vi "滑移力检测.vi"() -> ()   [LabVIEW 2020]
uses:
  <vilib>/Utility/config.llb/NI_LVConfig.lvlib
  Global_Variable/Global.vi
  Global_Variable/A131258.vi
  Database/Global1.vi
  <vilib>/addons/database/NI_Database_API.lvlib
  <vilib>/addons/database/Connection.llb/Conn Execute.vi
  <vilib>/addons/database/Recordset.llb/Rec Fetch Recordset Data (R).vi
  <vilib>/addons/database/Connection.llb/DB Tools Open Connec (String).vi
panel:
  out "Fdeviceid":string
  out "拉位移内最大压力追溯结果":bool
  out "压位移内最大压力追溯结果":bool
  out "USER_ID":string
  out "deviceid":string
  out "productid":string
  out "产品型号":string
  out "codeid":string
  out "联机模式":string
  out "用户权限":string
  out "用户名":string
  out "最小值下限":dbl format="%_4g"
  out "最小值上限":dbl format="%_4g"
  out "拉位移内最小压力(N)":dbl format="%_5g"
  out "压位移内最小压力(N)":dbl format="%_5g"
  in  "报表":string[][](table)=[["mm"], ["mm/s"]]
  in  "判定结果 3":bool[][](array[boolean])=[[TRUE]]
  out "拉力判定框内波动压力(N)":dbl format="%_5g"
  out "压力判定框内波动压力(N)":dbl format="%_5g"
  in  "选项卡控件 2":enum32{"滑移力曲线", "参数查看"}(tab)
  out "上序状态显示":string
  out "上序状态":bool
  in  "质量报警":bool
  in  "设备缺料":bool
  in  "设备故障":bool
  out "产品追溯码":string
  out "最大值下限":dbl format="%_4g"
  out "最大值上限":dbl format="%_4g"
  out "拉位移内最大压力(N)":dbl format="%_5g"
  out "压位移内最大压力(N)":dbl format="%_5g"
  out "合格指示灯":bool
  out "不合格指示灯":bool
  out "力位移曲线 3":cluster{dbl[], dbl[]}[](graph)
  in  "删除":bool
  in  "确定":bool
  in  "添加":bool
  in  "退出":bool
  in  "更新":bool
  in  "产品型号":string(combo)
  in  "选项卡控件 3":enum32{"工位参数", "产品管理", "用户管理"}(tab)
  in  "坐标轴参数":string[][](table)=[["mm"], ["mm/s"]]
  in  "判定框参数":string[][](table)=[["mm"], ["mm/s"]]
  in  "结果判定参数":string[][](table)=[["mm"], ["mm/s"]]
  in  "请输入添加的产品名称":string
  in  "请选择要删除的产品":string(combo)
  in  "进入用户管理":bool
  # "滑移力检测"
  # "上序状态："
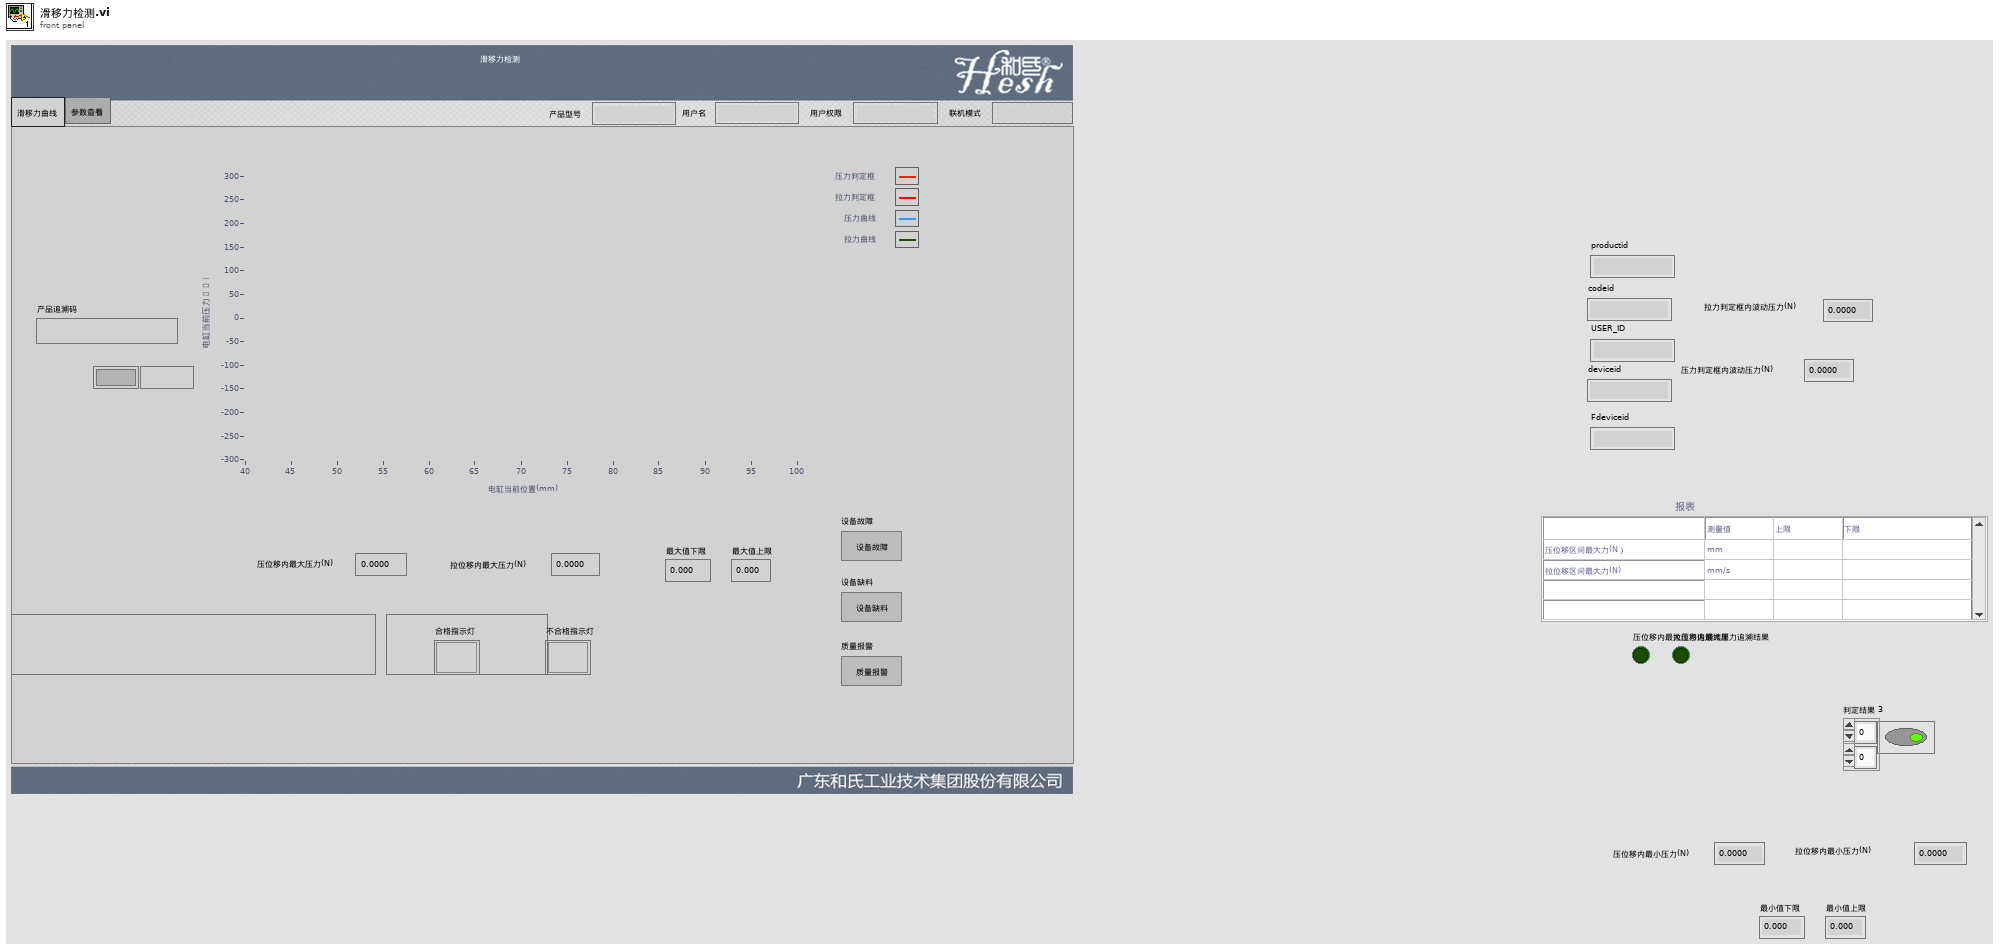
[diagram p1: front panel]
types:
  T1 = enum32{"Invalid", "Standard", "Closed", "Hidden", "Minimized", "Maximized"}
  T2 = cluster{"用户编号":string, "用户名":string, "用户密码(密文)":string, "用户权限":string}
  T3 = cluster{"设备名称":string, "用户名":string, "设备状态":enum16{"设备离线", "设备正常", "设备缺料", "设备故障", "质量报警"}, "附加信息":string}
  T4 = typedef "NI_LVConfig.lvlib/Config Data RefNum.ctl" = refnum<k1>
  T5 = cluster{i64, i64, string, "拉位移内最大压力(N)":dbl, "最大值下限":dbl, "最大值上限":dbl, string, string}
  T6 = cluster{i64, i64, string, "压位移内最大压力(N)":dbl, "最大值下限":dbl, "最大值上限":dbl, string, string}
  T7 = cluster{i64, i64, string, "拉位移内最大压力(N)":dbl, "最大值下限":dbl, "最大值上限":dbl, string, string}[]
  T8 = typedef "NI_Database_API.lvlib/Conn ObjectReference.ctl" = refnum<k1>
  T9 = cluster{i64, i64, "拉位移内最大压力(N)":dbl, "最大值下限":dbl, "最大值上限":dbl, string, string}
  T10 = cluster{i64, i64, i64, string, "result string":string}
  T11 = cluster{i64, i64, i64, string, "result string":string}[]
  T12 = typedef "NI_Database_API.lvlib/Rec ObjectReference.ctl" = refnum<k1>
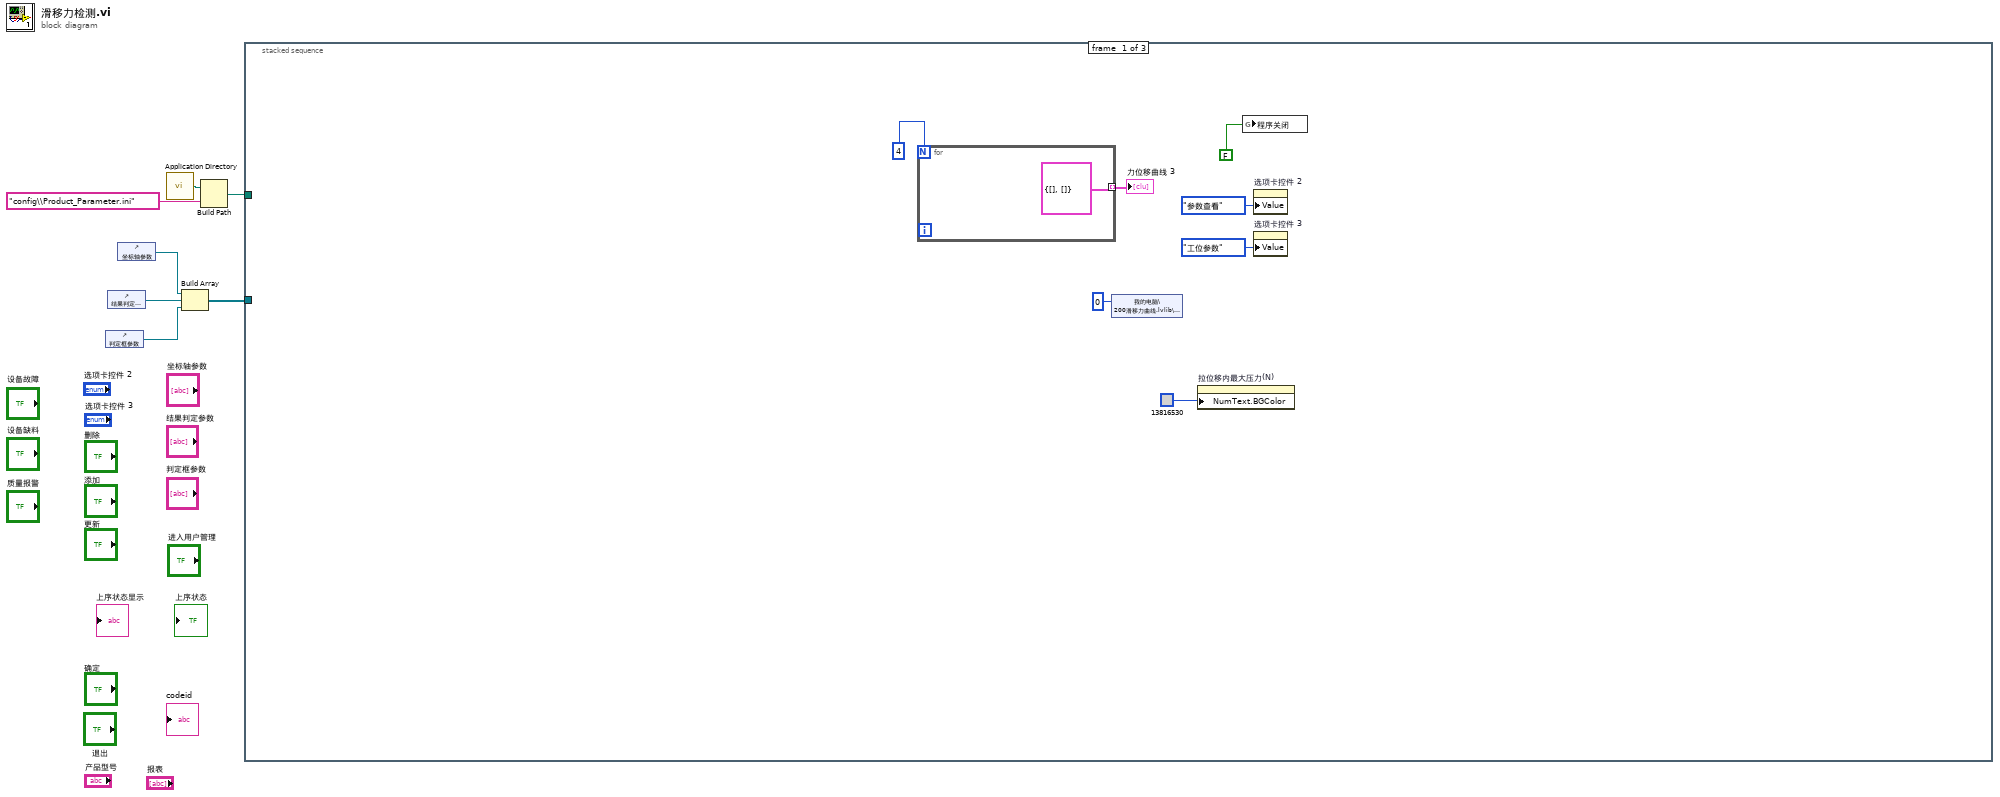
[diagram p0: block diagram]
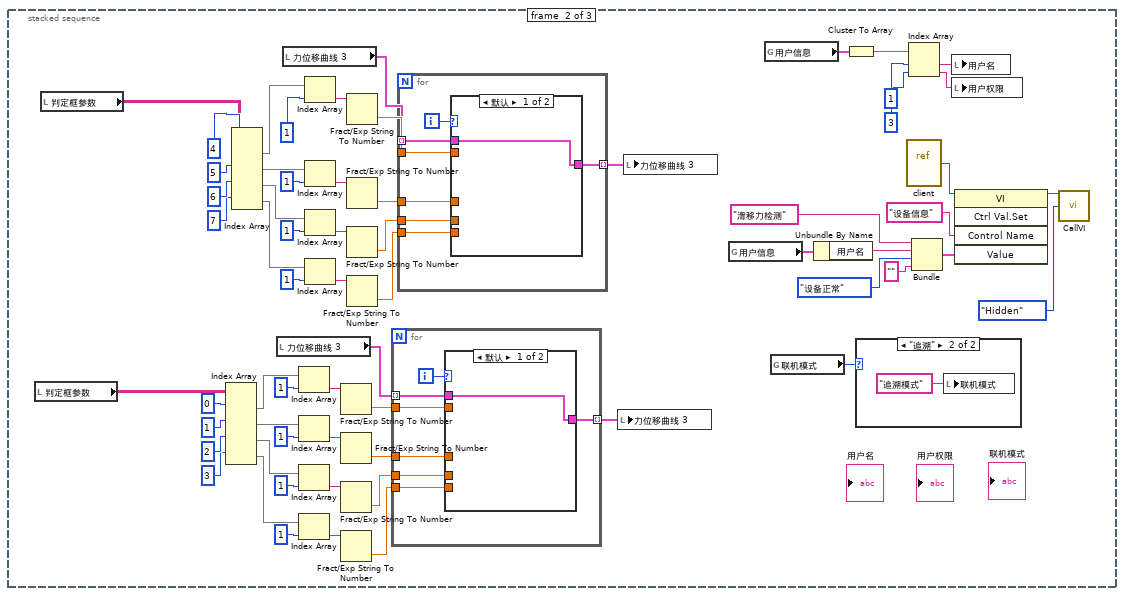
[diagram p2: hidden frame]
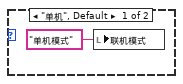
[diagram p3: hidden frame]
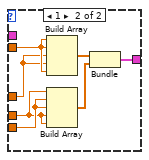
[diagram p4: hidden frame]
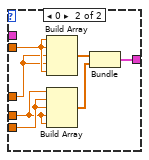
[diagram p5: hidden frame]
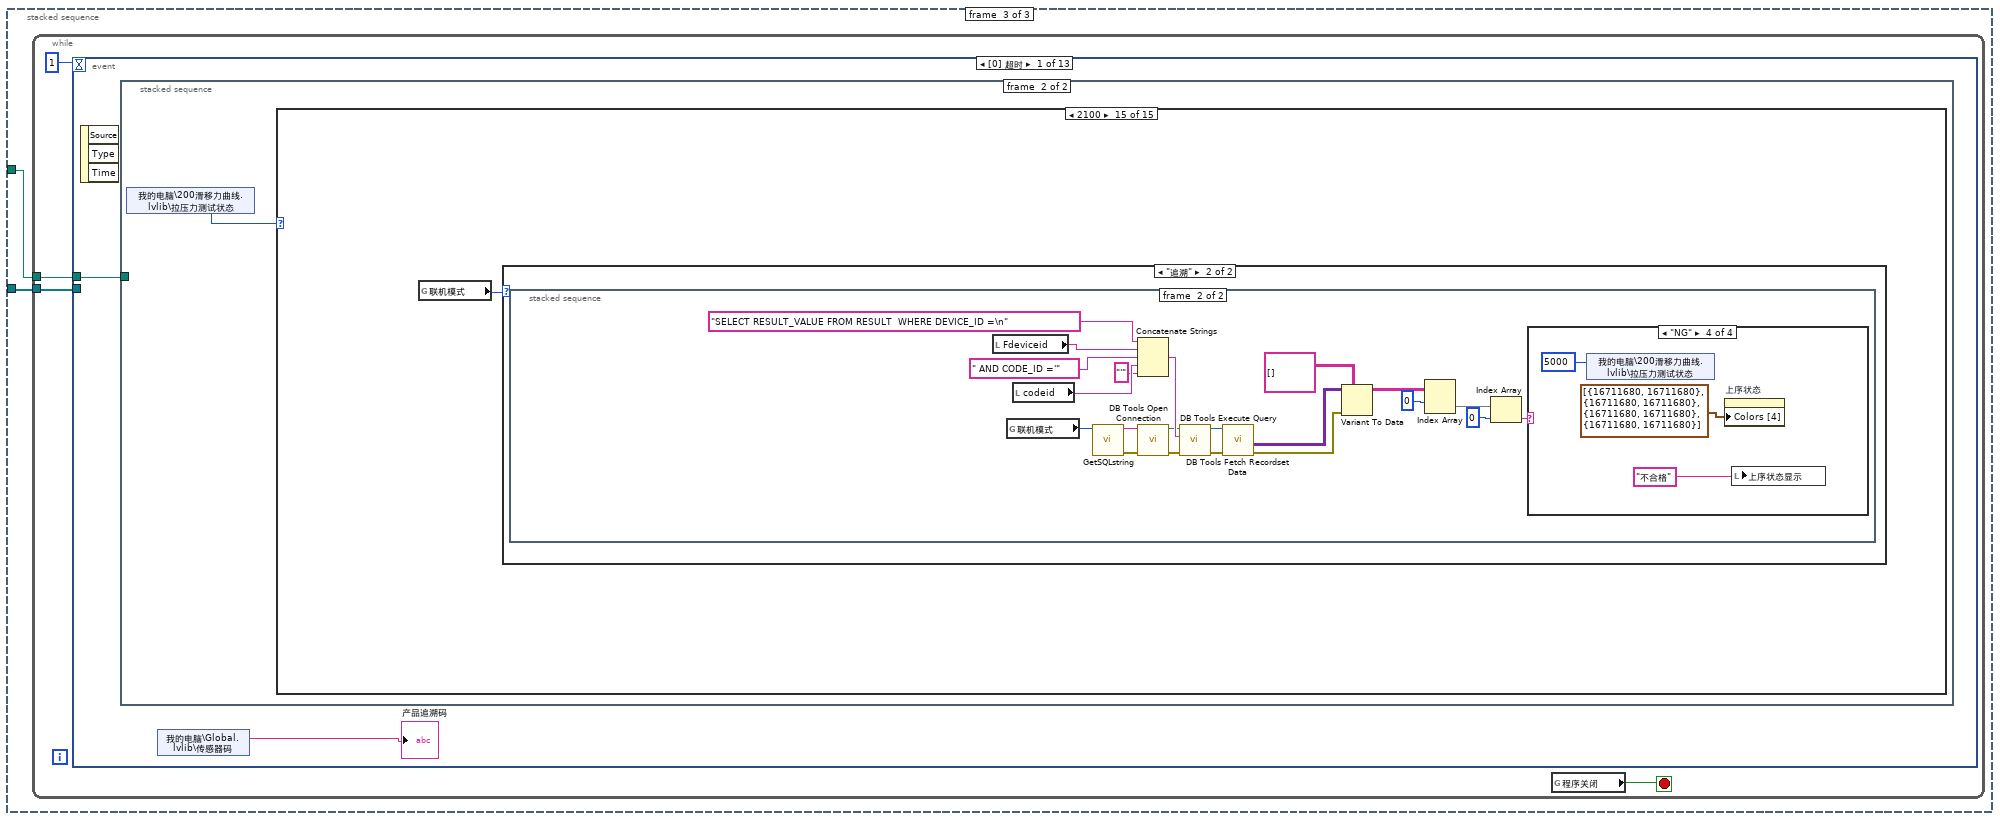
[diagram p6: hidden frame]
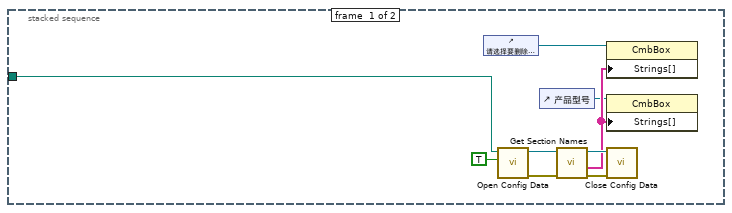
[diagram p7: hidden frame]
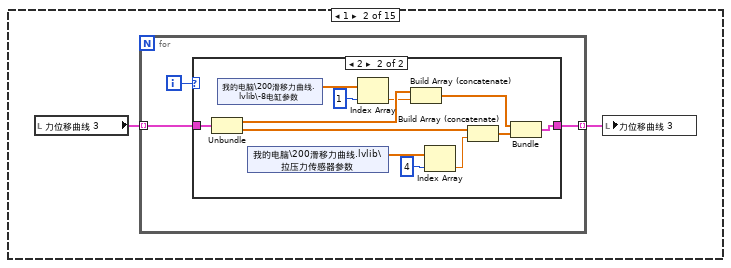
[diagram p9: hidden frame]
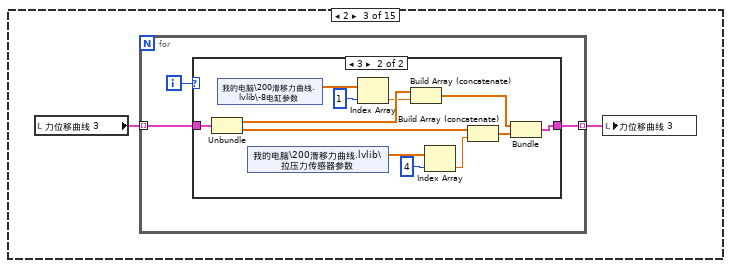
[diagram p11: hidden frame]
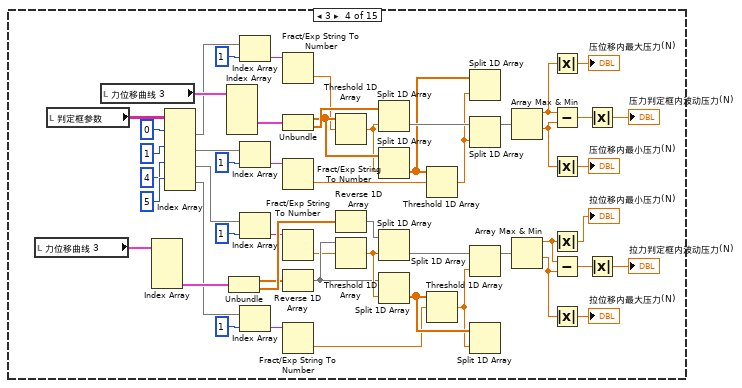
[diagram p13: hidden frame]
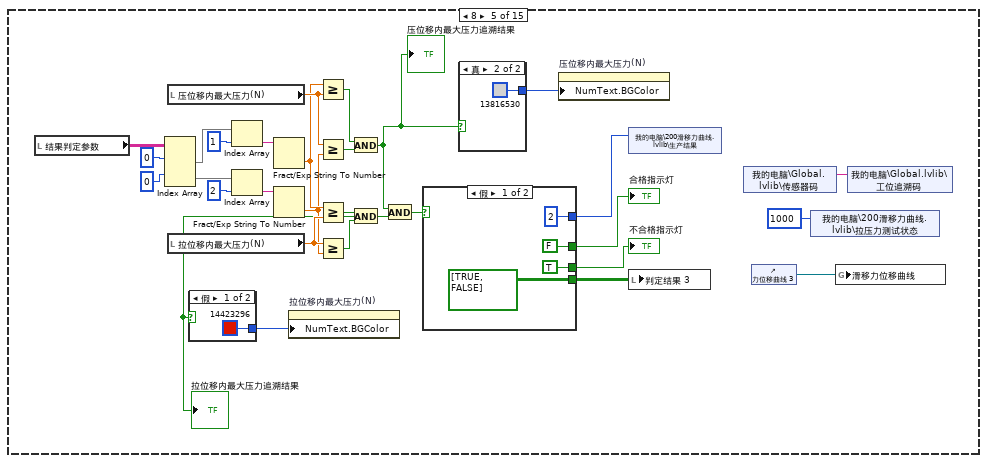
[diagram p14: hidden frame]
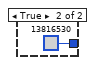
[diagram p15: hidden frame]
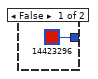
[diagram p16: hidden frame]
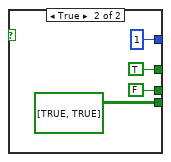
[diagram p17: hidden frame]
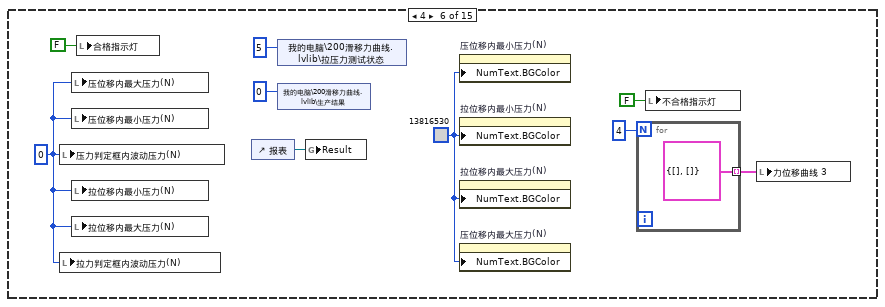
[diagram p18: hidden frame]
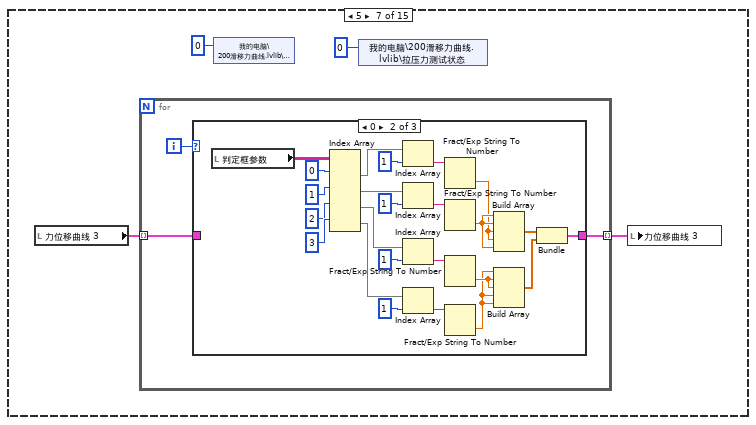
[diagram p19: hidden frame]
diagram:
  n1 = control-ref of="判定框参数"() -> (w1:refnum<vi>)
  n2 = control-ref of="结果判定参数"() -> (w2:refnum<vi>)
  n3 = control-ref of="坐标轴参数"() -> (w3:refnum<vi>)
  n4 = call <vilib>:"Application Directory.vi"() -> ("Application Directory"=w7:path)
  n5 = Build Array(w3, w2, w1) -> (w4:refnum<vi>[])
  n6 = Build Path(base path=w7, name or relative path="config\\Product_Parameter.ini" ("名称或相对路径")) -> (appended path=w5:path)
  n7 = stacked-sequence {
    tunnel: w5 -> [_ _ w112]
    tunnel: w4 -> [_ _ w111]
    frame #0 {
      n8 = for {
        N: 4 -> [_]
        tunnel: [cluster{dbl[], dbl[]} {[], []}] -> w13 mode=indexing
      }
      "力位移曲线 3" <- w13
      n9 = shared-variable "我的电脑\\200滑移力曲线.lvlib\\备用_1"(u16 0 ("备用_1")) -> ()  [unwired: 1 in, 1 out]
      n10 = property on="拉位移内最大压力(N)" class="DigNum (严格)"("NumText.BGColor"=u32 13816530) -> ()  [unwired: 2 in, 2 out]
      n11 = global write "Global.vi" "程序关闭"(FALSE ("程序关闭")) -> ()
      n12 = property on="选项卡控件 2" class="TabCtl (严格)"("Value"=enum32{"滑移力曲线", "参数查看"}."参数查看" ("选项卡控件 2")) -> ()  [unwired: 2 in, 2 out]
      n13 = property on="选项卡控件 3" class="TabCtl (严格)"("Value"=enum32{"工位参数", "产品管理"}."工位参数" ("选项卡控件 3")) -> ()  [unwired: 2 in, 2 out]
    }
    frame #1 {
      n14 = local read "判定框参数"() -> (w33:string[][])
      n15 = local read "判定框参数"() -> (w36:string[][])
      n16 = Index Array(array=w33, index (row) #1=0 ("索引 (行)"), index (row) #2=1 ("索引 (行)"), index (row) #3=2 ("索引 (行)"), index (row) #4=3 ("索引 (行)")) -> (element #1=w74:string[], element #2=w69:string[], element #3=w68:string[], element #4=w67:string[])  [unwired: 4 in]
      n17 = Index Array(array=w36, index (row) #1=4 ("索引 (行)"), index (row) #2=5 ("索引 (行)"), index (row) #3=6 ("索引 (行)"), index (row) #4=7 ("索引 (行)")) -> (element #1=w52:string[], element #2=w47:string[], element #3=w46:string[], element #4=w45:string[])  [unwired: 4 in]
      n18 = local read "力位移曲线 3"() -> (w57:cluster{dbl[], dbl[]}[])
      n19 = local read "力位移曲线 3"() -> (w35:cluster{dbl[], dbl[]}[])
      n20 = Index Array(array=w74, index=1 ("索引")) -> (element=w62:string)
      n21 = Index Array(array=w69, index=1 ("索引")) -> (element=w61:string)
      n22 = Index Array(array=w68, index=1 ("索引")) -> (element=w60:string)
      n23 = Index Array(array=w67, index=1 ("索引")) -> (element=w59:string)
      n24 = Index Array(array=w52, index=1 ("索引")) -> (element=w40:string)
      n25 = Index Array(array=w47, index=1 ("索引")) -> (element=w39:string)
      n26 = Index Array(array=w46, index=1 ("索引")) -> (element=w38:string)
      n27 = Index Array(array=w45, index=1 ("索引")) -> (element=w37:string)
      n28 = Fract/Exp String To Number(string=w62) -> (number=w66:dbl)  [unwired: 3 in, 1 out]
      n29 = Fract/Exp String To Number(string=w61) -> (number=w65:dbl)  [unwired: 3 in, 1 out]
      n30 = Fract/Exp String To Number(string=w60) -> (number=w63:dbl)  [unwired: 3 in, 1 out]
      n31 = Fract/Exp String To Number(string=w59) -> (number=w64:dbl)  [unwired: 3 in, 1 out]
      n32 = Fract/Exp String To Number(string=w40) -> (number=w44:dbl)  [unwired: 3 in, 1 out]
      n33 = Fract/Exp String To Number(string=w39) -> (number=w43:dbl)  [unwired: 3 in, 1 out]
      n34 = Fract/Exp String To Number(string=w38) -> (number=w41:dbl)  [unwired: 3 in, 1 out]
      n35 = Fract/Exp String To Number(string=w37) -> (number=w42:dbl)  [unwired: 3 in, 1 out]
      n36 = for {
        tunnel: [w102] -> w58 mode=indexing
        tunnel: w57 -> [w101] mode=indexing
        tunnel: w66 -> [w99]
        tunnel: w65 -> [w98]
        tunnel: w64 -> [w97]
        tunnel: w63 -> [w96]
        i -> [w100]
        n37 = case shown="默认" w100 {
          tunnel: [w103 w108] -> w102
          tunnel: w101 -> [w103 _]
          tunnel: w99 -> [_ w107]
          tunnel: w98 -> [_ w106]
          tunnel: w97 -> [_ w105]
          tunnel: w96 -> [_ w104]
          frame Default {
          }
          frame 0 {
            n38 = Build Array(w107, w107, w106, w106, w107) -> (w109:dbl[])
            n39 = Build Array(w104, w105, w105, w104, w104) -> (w110:dbl[])
            n40 = Bundle(w109, w110) -> (w108:cluster{dbl[], dbl[]})  [unwired: 1 in]
          }
        }
      }
      n41 = for {
        tunnel: [w87] -> w34 mode=indexing
        tunnel: w35 -> [w86] mode=indexing
        tunnel: w44 -> [w84]
        tunnel: w43 -> [w83]
        tunnel: w42 -> [w82]
        tunnel: w41 -> [w81]
        i -> [w85]
        n42 = case shown="默认" w85 {
          tunnel: [w88 w93] -> w87
          tunnel: w86 -> [w88 _]
          tunnel: w84 -> [_ w92]
          tunnel: w83 -> [_ w91]
          tunnel: w82 -> [_ w90]
          tunnel: w81 -> [_ w89]
          frame Default {
          }
          frame 1 {
            n43 = Build Array(w92, w92, w91, w91, w92) -> (w94:dbl[])
            n44 = Build Array(w89, w90, w90, w89, w89) -> (w95:dbl[])
            n45 = Bundle(w94, w95) -> (w93:cluster{dbl[], dbl[]})  [unwired: 1 in]
          }
        }
      }
      n46 = local write "力位移曲线 3"(w58) -> ()
      n47 = local write "力位移曲线 3"(w34) -> ()
      n48 = global read "Global1.vi" "用户信息"() -> (w23:T2)
      n49 = global read "Global1.vi" "用户信息"() -> (w32:T2)
      n50 = global read "Global1.vi" "联机模式"() -> (w26:enum16{"单机", "追溯"})
      n51 = Unbundle By Name(w23) -> ("用户名"=w22:string)
      n52 = Cluster To Array(cluster=w32) -> (array=w31:string[])
      n53 = case shown="\"追溯\"" w26 {
        frame "单机", Default {
          n54 = local write "联机模式"("单机模式" ("联机模式")) -> ()
        }
        frame "追溯" {
          n55 = local write "联机模式"("追溯模式" ("联机模式")) -> ()
        }
      }
      n56 = vi-ref "client.vi"() -> (w25:refnum<vi>)
      n57 = Index Array(array=w31, index #1=1 ("索引"), index #2=3 ("索引")) -> (element #1=w28:string, element #2=w27:string)
      n58 = Bundle("设备名称"="滑移力检测", "用户名"=w22, "设备状态"=enum16{"设备离线", "设备正常", "设备缺料", "设备故障", "质量报警"}."设备正常", "附加信息"="") -> (w21:T3)  [unwired: 1 in]
      n59 = local write "用户名"(w28) -> ()
      n60 = local write "用户权限"(w27) -> ()
      n61 = invoke class="VI" method="Ctrl Val.Set"(reference=w25, "Control Name"="设备信息" ("控件名"), "Value"=w21) -> (reference out=w24:refnum<vi>)  [unwired: 2 in, 4 out]
      n62 = call "CallVI.vi"("VI引用"=w24, "状态"=T1."Hidden") -> ()  [unwired: 11 in, 3 out]
    }
    frame #2 {
      n63 = while {
        tunnel: w112 -> [w115]
        tunnel: w111 -> [w114]
        stop <- w113 stop-if-true
        n64 = event shown="[0] 超时" {
          selector: _ -> [_ _ _ _ _ _ _ _ _ _ _ _ _]
          dyn-events: _ -> [_ _ _ _ _ _ _ _ _ _ _ _ _]
          timeout: 1 -> [_ _ _ _ _ _ _ _ _ _ _ _ _]
          tunnel: w115 -> [w118 w579 _ w747 w766 _ w777 _ _ _ _ _ _]
          tunnel: w114 -> [_ _ _ w746 w765 _ w776 _ _ _ _ _ _]
          event Timeout {
            n65 = event-data() -> ()  [unwired: 1 in, 3 out]
            n66 = stacked-sequence {
              tunnel: w118 -> [w119 _]
              frame #0 {
                n67 = control-ref of="请选择要删除的产品"() -> (w120:refnum<vi>)
                n68 = call <vilib>:"Open Config Data.vi"("create file if necessary (T)"=TRUE, "configuration file path"=w119) -> ("error out"=w124:errorcluster, "refnum"=w123:T4)  [unwired: 7 in, 1 out]
                n69 = control-ref of="产品型号"() -> (w121:refnum<vi>)
                n70 = call <vilib>:"Get Section Names.vi"("error in (no error)"=w124, "refnum"=w123) -> ("error out"=w126:errorcluster, "section names"=w122:string[], "refnum out"=w125:T4)  [unwired: 7 in]
                n71 = property on="属性节点" class="CmbBox"(reference=w120, "Strings[]"=w122) -> ()  [unwired: 1 in, 2 out]
                n72 = property on="属性节点" class="CmbBox"(reference=w121, "Strings[]"=w122) -> ()  [unwired: 1 in, 2 out]
                n73 = call <vilib>:"Close Config Data.vi"("error in (no error)"=w126, "refnum"=w125) -> ()  [unwired: 8 in, 2 out]
              }
              frame #1 {
                n74 = shared-variable "我的电脑\\200滑移力曲线.lvlib\\拉压力测试状态"() -> (w128:u16)  [unwired: 1 in, 1 out]
                n75 = case shown="2100" w128 {
                  frame 0, Default {
                  }
                  frame 1 {
                    n76 = local read "力位移曲线 3"() -> (w129:cluster{dbl[], dbl[]}[])
                    n77 = for {
                      tunnel: [w133] -> w130 mode=indexing
                      tunnel: w129 -> [w132] mode=indexing
                      i -> [w131]
                      n78 = case shown="2" w131 {
                        tunnel: [w134 w140] -> w133
                        tunnel: w132 -> [w134 w139]
                        frame Default {
                        }
                        frame 2 {
                          n79 = Unbundle(w139) -> (w144:dbl[], w143:dbl[])
                          n80 = shared-variable "我的电脑\\200滑移力曲线.lvlib\\-8电缸参数"() -> (w135:sgl[])  [unwired: 1 in, 1 out]
                          n81 = shared-variable "我的电脑\\200滑移力曲线.lvlib\\拉压力传感器参数"() -> (w136:sgl[])  [unwired: 1 in, 1 out]
                          n82 = Index Array(array=w135, index=1) -> (element=w137:sgl)
                          n83 = Build Array (concatenate)(w144, w137) -> (w142:dbl[])
                          n84 = Index Array(array=w136, index=4) -> (element=w138:sgl)
                          n85 = Build Array (concatenate)(w143, w138) -> (w141:dbl[])
                          n86 = Bundle(w142, w141) -> (w140:cluster{dbl[], dbl[]})  [unwired: 1 in]
                        }
                      }
                    }
                    n87 = local write "力位移曲线 3"(w130) -> ()
                  }
                  frame 2 {
                    n88 = local read "力位移曲线 3"() -> (w147:cluster{dbl[], dbl[]}[])
                    n89 = for {
                      tunnel: [w151] -> w148 mode=indexing
                      tunnel: w147 -> [w150] mode=indexing
                      i -> [w149]
                      n90 = case shown="3" w149 {
                        tunnel: [w152 w158] -> w151
                        tunnel: w150 -> [w152 w157]
                        frame Default {
                        }
                        frame 3 {
                          n91 = Unbundle(w157) -> (w162:dbl[], w161:dbl[])
                          n92 = shared-variable "我的电脑\\200滑移力曲线.lvlib\\-8电缸参数"() -> (w153:sgl[])  [unwired: 1 in, 1 out]
                          n93 = shared-variable "我的电脑\\200滑移力曲线.lvlib\\拉压力传感器参数"() -> (w154:sgl[])  [unwired: 1 in, 1 out]
                          n94 = Index Array(array=w153, index=1) -> (element=w155:sgl)
                          n95 = Build Array (concatenate)(w162, w155) -> (w160:dbl[])
                          n96 = Index Array(array=w154, index=4) -> (element=w156:sgl)
                          n97 = Build Array (concatenate)(w161, w156) -> (w159:dbl[])
                          n98 = Bundle(w160, w159) -> (w158:cluster{dbl[], dbl[]})  [unwired: 1 in]
                        }
                      }
                    }
                    n99 = local write "力位移曲线 3"(w148) -> ()
                  }
                  frame 3 {
                    n100 = local read "力位移曲线 3"() -> (w209:cluster{dbl[], dbl[]}[])
                    n101 = local read "判定框参数"() -> (w177:string[][])
                    n102 = local read "力位移曲线 3"() -> (w217:cluster{dbl[], dbl[]}[])
                    n103 = Index Array(array=w209) -> (element #4=w202:cluster{dbl[], dbl[]})  [unwired: 4 in, 3 out]
                    n104 = Index Array(array=w177, index (row) #1=0 ("索引 (行)"), index (row) #2=1 ("索引 (行)"), index (row) #3=4 ("索引 (行)"), index (row) #4=5 ("索引 (行)")) -> (element #1=w169:string[], element #2=w170:string[], element #3=w171:string[], element #4=w172:string[])  [unwired: 4 in]
                    n105 = Index Array(array=w217) -> (element #3=w203:cluster{dbl[], dbl[]})  [unwired: 4 in, 3 out]
                    n106 = Unbundle(w202) -> (w187:dbl[], w189:dbl[])
                    n107 = Index Array(array=w169, index=1 ("索引")) -> (element=w173:string)
                    n108 = Index Array(array=w170, index=1 ("索引")) -> (element=w174:string)
                    n109 = Index Array(array=w171, index=1 ("索引")) -> (element=w175:string)
                    n110 = Index Array(array=w172, index=1 ("索引")) -> (element=w176:string)
                    n111 = Fract/Exp String To Number(string=w173) -> (number=w168:dbl)  [unwired: 3 in, 1 out]
                    n112 = Unbundle(w203) -> (w215:dbl[], w216:dbl[])
                    n113 = Fract/Exp String To Number(string=w174) -> (number=w167:dbl)  [unwired: 3 in, 1 out]
                    n114 = Fract/Exp String To Number(string=w175) -> (number=w166:dbl)  [unwired: 3 in, 1 out]
                    n115 = Reverse 1D Array(array=w187) -> (reversed array=w186:dbl[])
                    n116 = Fract/Exp String To Number(string=w176) -> (number=w165:dbl)  [unwired: 3 in, 1 out]
                    n117 = Threshold 1D Array(2:w168, 3:w215) -> (0:w214:dbl)  [unwired: 1 in]
                    n118 = Reverse 1D Array(array=w189) -> (reversed array=w188:dbl[])
                    n119 = Threshold 1D Array(2:w166, 3:w186) -> (0:w208:dbl)  [unwired: 1 in]
                    n120 = Split 1D Array(array=w216, index=w214) -> (second subarray=w213:dbl[])  [unwired: 1 out]
                    n121 = Split 1D Array(array=w215, index=w214) -> (second subarray=w212:dbl[])  [unwired: 1 out]
                    n122 = Split 1D Array(array=w188, index=w208) -> (second subarray=w207:dbl[])  [unwired: 1 out]
                    n123 = Split 1D Array(array=w186, index=w208) -> (second subarray=w206:dbl[])  [unwired: 1 out]
                    n124 = Threshold 1D Array(2:w167, 3:w212) -> (0:w211:dbl)  [unwired: 1 in]
                    n125 = Threshold 1D Array(2:w165, 3:w206) -> (0:w205:dbl)  [unwired: 1 in]
                    n126 = Split 1D Array(array=w212, index=w211) -> ()  [unwired: 2 out]
                    n127 = Split 1D Array(array=w213, index=w211) -> (first subarray=w210:dbl[])  [unwired: 1 out]
                    n128 = Split 1D Array(array=w207, index=w205) -> (first subarray=w204:dbl[])  [unwired: 1 out]
                    n129 = Split 1D Array(array=w206, index=w205) -> ()  [unwired: 2 out]
                    n130 = Array Max & Min(array=w210) -> (max value=w193:dbl, min value=w191:dbl)  [unwired: 2 out]
                    n131 = Array Max & Min(array=w204) -> (max value=w201:dbl, min value=w199:dbl)  [unwired: 2 out]
                    n132 = Absolute Value(x=w193) -> (abs(x)=→"压位移内最大压力(N)":dbl)
                    n133 = Subtract(x=w193, y=w191) -> (x-y=w195:dbl)
                    n134 = Absolute Value(x=w191) -> (abs(x)=→"压位移内最小压力(N)":dbl)
                    n135 = Absolute Value(x=w201) -> (abs(x)=→"拉位移内最小压力(N)":dbl)
                    n136 = Subtract(x=w201, y=w199) -> (x-y=w197:dbl)
                    n137 = Absolute Value(x=w199) -> (abs(x)=→"拉位移内最大压力(N)":dbl)
                    n138 = Absolute Value(x=w195) -> (abs(x)=→"压力判定框内波动压力(N)":dbl)
                    n139 = Absolute Value(x=w197) -> (abs(x)=→"拉力判定框内波动压力(N)":dbl)
                  }
                  frame 8 {
                    n140 = local read "结果判定参数"() -> (w233:string[][])
                    n141 = Index Array(array=w233, index (row) #1=0 ("索引 (行)"), index (row) #2=0 ("索引 (行)")) -> (element #1=w229:string[], element #2=w230:string[])  [unwired: 2 in]
                    n142 = local read "压位移内最大压力(N)"() -> (w242:dbl)
                    n143 = local read "拉位移内最大压力(N)"() -> (w241:dbl)
                    n144 = Index Array(array=w229, index=1 ("索引")) -> (element=w231:string)
                    n145 = Index Array(array=w230, index=2 ("索引")) -> (element=w232:string)
                    n146 = Fract/Exp String To Number(string=w231) -> (number=w228:dbl)  [unwired: 3 in, 1 out]
                    n147 = Fract/Exp String To Number(string=w232) -> (number=w227:dbl)  [unwired: 3 in, 1 out]
                    n148 = Greater Or Equal?(x=w228, y=w242) -> (x >= y?=w246:bool)
                    n149 = Greater Or Equal?(x=w242, y=w227) -> (x >= y?=w245:bool)
                    n150 = Greater Or Equal?(x=w228, y=w241) -> (x >= y?=w244:bool)
                    n151 = Greater Or Equal?(x=w241, y=w227) -> (x >= y?=w243:bool)
                    n152 = And(x=w246, y=w245) -> (x .and. y?=w219:bool)
                    "压位移内最大压力追溯结果" <- w219
                    n153 = And(x=w244, y=w243) -> (x .and. y?=w218:bool)
                    "拉位移内最大压力追溯结果" <- w218
                    n154 = case shown="假" w218 {
                      tunnel: [u32 14423296 u32 13816530] -> w225
                      frame False {
                      }
                      frame True {
                      }
                    }
                    n155 = property on="拉位移内最大压力(N)" class="DigNum (严格)"("NumText.BGColor"=w225) -> ()  [unwired: 2 in, 2 out]
                    n156 = And(x=w219, y=w218) -> (x .and. y?=w220:bool)
                    n157 = case shown="假" w220 {
                      tunnel: [u16 2 ("生产结果") u16 1 ("生产结果")] -> w240
                      tunnel: [FALSE ("合格指示灯") TRUE ("合格指示灯")] -> w239
                      tunnel: [TRUE ("不合格指示灯") FALSE ("不合格指示灯")] -> w238
                      tunnel: [bool[][] [[TRUE, FALSE]] ("判定结果") bool[][] [[TRUE, TRUE]] ("判定结果")] -> w224
                      frame False {
                      }
                      frame True {
                      }
                    }
                    "不合格指示灯" <- w238
                    "合格指示灯" <- w239
                    n158 = case shown="真" w219 {
                      tunnel: [u32 14423296 u32 13816530] -> w226
                      frame False {
                      }
                      frame True {
                      }
                    }
                    n159 = property on="压位移内最大压力(N)" class="DigNum (严格)"("NumText.BGColor"=w226) -> ()  [unwired: 2 in, 2 out]
                    n160 = shared-variable "我的电脑\\200滑移力曲线.lvlib\\生产结果"(w240) -> ()  [unwired: 1 in, 1 out]
                    n161 = local write "判定结果 3"(w224) -> ()
                    n162 = shared-variable "我的电脑\\Global.lvlib\\传感器码"() -> (w223:string)  [unwired: 1 in, 1 out]
                    n163 = control-ref of="力位移曲线 3"() -> (w221:refnum<vi>)
                    n164 = shared-variable "我的电脑\\200滑移力曲线.lvlib\\拉压力测试状态"(u16 1000 ("拉压力测试状态")) -> ()  [unwired: 1 in, 1 out]
                    n165 = global write "A131258.vi" "滑移力位移曲线"(w221) -> ()
                    n166 = shared-variable "我的电脑\\Global.lvlib\\工位追溯码"(w223) -> ()  [unwired: 1 in, 1 out]
                  }
                  frame 4 {
                    w260 = u32 13816530
                    w264 = 0
                    n167 = local write "压力判定框内波动压力(N)"(w264) -> ()
                    n168 = local write "拉力判定框内波动压力(N)"(w264) -> ()
                    n169 = local write "压位移内最大压力(N)"(w264) -> ()
                    n170 = local write "压位移内最小压力(N)"(w264) -> ()
                    n171 = local write "拉位移内最小压力(N)"(w264) -> ()
                    n172 = local write "拉位移内最大压力(N)"(w264) -> ()
                    n173 = local write "合格指示灯"(FALSE ("合格指示灯")) -> ()
                    n174 = control-ref of="报表"() -> (w259:refnum<vi>)
                    n175 = shared-variable "我的电脑\\200滑移力曲线.lvlib\\拉压力测试状态"(5) -> ()  [unwired: 1 in, 1 out]
                    n176 = shared-variable "我的电脑\\200滑移力曲线.lvlib\\生产结果"(u16 0 ("生产结果")) -> ()  [unwired: 1 in, 1 out]
                    n177 = global write "Global.vi" "Result"(w259) -> ()
                    n178 = property on="压位移内最小压力(N)" class="DigNum (严格)"("NumText.BGColor"=w260) -> ()  [unwired: 2 in, 2 out]
                    n179 = property on="拉位移内最小压力(N)" class="DigNum (严格)"("NumText.BGColor"=w260) -> ()  [unwired: 2 in, 2 out]
                    n180 = property on="拉位移内最大压力(N)" class="DigNum (严格)"("NumText.BGColor"=w260) -> ()  [unwired: 2 in, 2 out]
                    n181 = property on="压位移内最大压力(N)" class="DigNum (严格)"("NumText.BGColor"=w260) -> ()  [unwired: 2 in, 2 out]
                    n182 = for {
                      N: 4 -> [_]
                      tunnel: [cluster{dbl[], dbl[]} {[], []}] -> w267 mode=indexing
                    }
                    n183 = local write "不合格指示灯"(FALSE ("不合格指示灯")) -> ()
                    n184 = local write "力位移曲线 3"(w267) -> ()
                  }
                  frame 5 {
                    n185 = local read "力位移曲线 3"() -> (w272:cluster{dbl[], dbl[]}[])
                    n186 = for {
                      tunnel: [w275] -> w271 mode=indexing
                      tunnel: w272 -> [w274] mode=indexing
                      i -> [w273]
                      n187 = case shown="0" w273 {
                        tunnel: [w276 w298 w301] -> w275
                        tunnel: w274 -> [w276 _ _]
                        frame Default {
                        }
                        frame 0 {
                          n188 = local read "判定框参数"() -> (w289:string[][])
                          n189 = Index Array(array=w289, index (row) #1=0 ("索引 (行)"), index (row) #2=1 ("索引 (行)"), index (row) #3=2 ("索引 (行)"), index (row) #4=3 ("索引 (行)")) -> (element #1=w281:string[], element #2=w282:string[], element #3=w283:string[], element #4=w284:string[])  [unwired: 4 in]
                          n190 = Index Array(array=w281, index=1 ("索引")) -> (element=w285:string)
                          n191 = Index Array(array=w282, index=1 ("索引")) -> (element=w286:string)
                          n192 = Index Array(array=w283, index=1 ("索引")) -> (element=w287:string)
                          n193 = Index Array(array=w284, index=1 ("索引")) -> (element=w288:string)
                          n194 = Fract/Exp String To Number(string=w285) -> (number=w279:dbl)  [unwired: 3 in, 1 out]
                          n195 = Fract/Exp String To Number(string=w286) -> (number=w280:dbl)  [unwired: 3 in, 1 out]
                          n196 = Fract/Exp String To Number(string=w287) -> (number=w278:dbl)  [unwired: 3 in, 1 out]
                          n197 = Fract/Exp String To Number(string=w288) -> (number=w277:dbl)  [unwired: 3 in, 1 out]
                          n198 = Build Array(w280, w280, w279, w279, w280) -> (w299:dbl[])
                          n199 = Build Array(w277, w278, w278, w277, w277) -> (w300:dbl[])
                          n200 = Bundle(w299, w300) -> (w298:cluster{dbl[], dbl[]})  [unwired: 1 in]
                        }
                        frame 1 {
                          n201 = local read "判定框参数"() -> (w322:string[][])
                          n202 = Index Array(array=w322, index (row) #1=4 ("索引 (行)"), index (row) #2=5 ("索引 (行)"), index (row) #3=6 ("索引 (行)"), index (row) #4=7 ("索引 (行)")) -> (element #1=w314:string[], element #2=w315:string[], element #3=w316:string[], element #4=w317:string[])  [unwired: 4 in]
                          n203 = Index Array(array=w314, index=1 ("索引")) -> (element=w318:string)
                          n204 = Index Array(array=w315, index=1 ("索引")) -> (element=w319:string)
                          n205 = Index Array(array=w316, index=1 ("索引")) -> (element=w320:string)
                          n206 = Index Array(array=w317, index=1 ("索引")) -> (element=w321:string)
                          n207 = Fract/Exp String To Number(string=w318) -> (number=w312:dbl)  [unwired: 3 in, 1 out]
                          n208 = Fract/Exp String To Number(string=w319) -> (number=w313:dbl)  [unwired: 3 in, 1 out]
                          n209 = Fract/Exp String To Number(string=w320) -> (number=w311:dbl)  [unwired: 3 in, 1 out]
                          n210 = Fract/Exp String To Number(string=w321) -> (number=w310:dbl)  [unwired: 3 in, 1 out]
                          n211 = Build Array(w313, w313, w312, w312, w313) -> (w323:dbl[])
                          n212 = Build Array(w310, w311, w311, w310, w310) -> (w324:dbl[])
                          n213 = Bundle(w323, w324) -> (w301:cluster{dbl[], dbl[]})  [unwired: 1 in]
                        }
                      }
                    }
                    n214 = shared-variable "我的电脑\\200滑移力曲线.lvlib\\备用_1"(u16 0 ("备用_1")) -> ()  [unwired: 1 in, 1 out]
                    n215 = shared-variable "我的电脑\\200滑移力曲线.lvlib\\拉压力测试状态"(0) -> ()  [unwired: 1 in, 1 out]
                    n216 = local write "力位移曲线 3"(w271) -> ()
                  }
                  frame 101 {
                    w327 = u32 13816530
                    w329 = 0.0 ("压力判定框内最大压力(N)")
                    w332 = FALSE ("合格指示灯")
                    n217 = shared-variable "我的电脑\\200滑移力曲线.lvlib\\备用_1"(u16 0 ("备用_1")) -> ()  [unwired: 1 in, 1 out]
                    n218 = local write "压位移内最大压力(N)"(w329) -> ()
                    n219 = local write "压位移内最小压力(N)"(w329) -> ()
                    n220 = local write "压力判定框内波动压力(N)"(w329) -> ()
                    n221 = local write "拉位移内最小压力(N)"(w329) -> ()
                    n222 = local write "拉位移内最大压力(N)"(w329) -> ()
                    n223 = local write "拉力判定框内波动压力(N)"(w329) -> ()
                    n224 = local write "合格指示灯"(w332) -> ()
                    n225 = local write "不合格指示灯"(w332) -> ()
                    n226 = property on="压位移内最大压力(N)" class="DigNum (严格)"("NumText.BGColor"=w327) -> ()  [unwired: 2 in, 2 out]
                    n227 = property on="压位移内最小压力(N)" class="DigNum (严格)"("NumText.BGColor"=w327) -> ()  [unwired: 2 in, 2 out]
                    n228 = property on="拉位移内最小压力(N)" class="DigNum (严格)"("NumText.BGColor"=w327) -> ()  [unwired: 2 in, 2 out]
                    n229 = property on="拉位移内最大压力(N)" class="DigNum (严格)"("NumText.BGColor"=w327) -> ()  [unwired: 2 in, 2 out]
                    n230 = shared-variable "我的电脑\\200滑移力曲线.lvlib\\生产结果"(u16 0 ("生产结果")) -> ()  [unwired: 1 in, 1 out]
                    n231 = shared-variable "我的电脑\\200滑移力曲线.lvlib\\拉压力测试状态"(0) -> ()  [unwired: 1 in, 1 out]
                    n232 = for {
                      N: 4 -> [_]
                      tunnel: [cluster{dbl[], dbl[]} {[], []}] -> w331 mode=indexing
                    }
                    n233 = local write "力位移曲线 3"(w331) -> ()
                  }
                  frame 1000 {
                    n234 = local read "压位移内最大压力(N)"() -> (w353:dbl)
                    n235 = local read "拉位移内最大压力(N)"() -> (w352:dbl)
                    n236 = local read "最大值上限"() -> (w350:dbl)
                    n237 = local read "最大值下限"() -> (w349:dbl)
                    n238 = local read "最大值上限"() -> (w348:dbl)
                    n239 = local read "最大值下限"() -> (w347:dbl)
                    n240 = Number To Fractional String(number=w353, precision (6)=i16 3 ("精度(6)")) -> (F-format string=w357:string)  [unwired: 2 in]
                    n241 = Number To Fractional String(number=w350, precision (6)=i16 3 ("精度(6)")) -> (F-format string=w356:string)  [unwired: 2 in]
                    n242 = Number To Fractional String(number=w349, precision (6)=i16 3 ("精度(6)")) -> (F-format string=w354:string)  [unwired: 2 in]
                    n243 = Number To Fractional String(number=w352, precision (6)=i16 3 ("精度(6)")) -> (F-format string=w351:string)  [unwired: 2 in]
                    n244 = Number To Fractional String(number=w348, precision (6)=i16 3 ("精度(6)")) -> (F-format string=w346:string)  [unwired: 2 in]
                    n245 = Number To Fractional String(number=w347, precision (6)=i16 3 ("精度(6)")) -> (F-format string=w345:string)  [unwired: 2 in]
                    n246 = Build Array(w357, w356, w354) -> (w355:string[])
                    n247 = Build Array(w351, w346, w345) -> (w335:string[])
                    n248 = Build Array(w355, w335) -> (w344:string[][])
                    n249 = local write "报表"(w344) -> ()
                    n250 = stacked-sequence {
                      frame #0 {
                        n251 = Wait (ms)(milliseconds to wait=u32 500 ("等待时间（毫秒）")) -> ()  [unwired: 1 out]
                        n252 = call "浮动通知.vi"("通知内容"="报表生成中" ("Status")) -> ()  [unwired: 11 in]
                      }
                      frame #1 {
                      }
                    }
                    n253 = control-ref of="报表"() -> (w343:refnum<vi>)
                    n254 = shared-variable "我的电脑\\200滑移力曲线.lvlib\\拉压力测试状态"(u16 1001 ("拉压力测试状态")) -> ()  [unwired: 1 in, 1 out]
                    n255 = shared-variable "我的电脑\\200滑移力曲线.lvlib\\备用_1"(u16 1 ("备用_1")) -> ()  [unwired: 1 in, 1 out]
                    n256 = global write "Global.vi" "Result"(w343) -> ()
                  }
                  frame 1001 {
                    n257 = shared-variable "我的电脑\\Global.lvlib\\工位追溯码"() -> (w364:string)  [unwired: 1 in, 1 out]
                    n258 = Wait (ms)(milliseconds to wait=u32 800 ("等待时间（毫秒）")) -> ()  [unwired: 1 out]
                    n259 = call "Report_A131258.vi"("文件重命名"=TRUE, "文件名称"=w364, "布尔数组"="判定结果 3") -> ()  [unwired: 8 in, 1 out]
                    n260 = shared-variable "我的电脑\\200滑移力曲线.lvlib\\拉压力测试状态"(u16 1002 ("备用1")) -> ()  [unwired: 1 in, 1 out]
                  }
                  frame 1002 {
                    n261 = global read "Global1.vi" "联机模式"() -> (w365:enum16{"单机", "追溯"})
                    n262 = case shown="\"追溯\"" w365 {
                      tunnel: w365 -> [_ w367]
                      frame "单机", Default {
                        n263 = shared-variable "我的电脑\\200滑移力曲线.lvlib\\拉压力测试状态"(u16 1003 ("备用1")) -> ()  [unwired: 1 in, 1 out]
                      }
                      frame "追溯" {
                        n264 = stacked-sequence {
                          tunnel: w367 -> [w368 _]
                          frame #0 {
                            n265 = local read "拉位移内最大压力追溯结果"() -> (w369:bool)
                            n266 = local read "压位移内最大压力追溯结果"() -> (w372:bool)
                            n267 = local read "拉位移内最大压力(N)"() -> (w382:dbl)
                            n268 = local read "压位移内最大压力(N)"() -> (w387:dbl)
                            n269 = local read "deviceid"() -> (w378:string)
                            n270 = local read "deviceid"() -> (w393:string)
                            n271 = local read "codeid"() -> (w381:string)
                            n272 = local read "codeid"() -> (w389:string)
                            n273 = local read "最大值下限"() -> (w383:dbl)
                            n274 = local read "最大值上限"() -> (w384:dbl)
                            n275 = local read "最大值下限"() -> (w386:dbl)
                            n276 = local read "最大值上限"() -> (w385:dbl)
                            n277 = case shown="假" w372 {
                              tunnel: ["NG" "OK"] -> w371
                              frame False {
                              }
                              frame True {
                              }
                            }
                            n278 = case shown="假" w369 {
                              tunnel: ["NG" "OK"] -> w370
                              frame False {
                              }
                              frame True {
                              }
                            }
                            n279 = Decimal String To Number(string=w378, default (0L)=i64 0 ("默认(0 I32)")) -> (number=w379:i64)  [unwired: 1 in, 1 out]
                            n280 = Decimal String To Number(string=w393, default (0L)=i64 0 ("默认(0 I32)")) -> (number=w391:i64)  [unwired: 1 in, 1 out]
                            n281 = Decimal String To Number(string=w381, default (0L)=i64 0 ("默认(0 I32)")) -> (number=w380:i64)  [unwired: 1 in, 1 out]
                            n282 = Decimal String To Number(string=w389, default (0L)=i64 0 ("默认(0 I32)")) -> (number=w390:i64)  [unwired: 1 in, 1 out]
                            n283 = Bundle(w379, w380, "拉位移内最大压力", "拉位移内最大压力(N)"=w382, "最大值下限"=w383, "最大值上限"=w384, "N", w370) -> (w373:T5)  [unwired: 1 in]
                            n284 = Bundle(w391, w390, "压位移内最大压力", "压位移内最大压力(N)"=w387, "最大值下限"=w386, "最大值上限"=w385, "N", w371) -> (w395:T6)  [unwired: 1 in]
                            n285 = Build Array(w395, w373) -> (w394:T7)
                            n286 = call "GetSQLstring.vi"("联机模式"=w368) -> ("错误输出"=w400:errorcluster, "连接字符串"=w401:string)  [unwired: 9 in]
                            n287 = call-poly <vilib>:"DB Tools Open Connection.vi"("error in (no error)"=w400, "connection information"=w401) -> ("error out"=w402:errorcluster, "connection reference"=w398:T8)  [unwired: 6 in]
                            n288 = for {
                              tunnel: w394 -> [w411] mode=indexing
                              tunnel: w398 -> [w409]
                              shift-right: [w407] -> w396
                              shift-left: w402 -> [w414]
                              w410 = string[] ["DEVICE_ID", "CODE_ID", "TEST_NAME", "TEST_VALUE", "TEST_VALUE_MIN", "TEST_VALUE_MAX", "TEST_VALUE_UNIT", "TEST_VALUE_RESULT"] ("columns")
                              w412 = "Test" ("table")
                              n289 = call <vilib>:"DB Tools Insert Data.vi"("data"=w411, "error in (no error)"=w414, "columns"=w410, "table"=w412, "connection reference"=w409) -> ("error out"=w413:errorcluster, "connection reference out"=w408:T8)  [unwired: 5 in]
                              n290 = case shown="错误" w413 {
                                selector: w413 -> [w415 w440]
                                tunnel: w410 -> [_ w437]
                                tunnel: w408 -> [w416 w422]
                                tunnel: w412 -> [_ w441]
                                tunnel: w411 -> [_ w431]
                                tunnel: [w416 w421] -> _
                                tunnel: [w415 w420] -> w407
                                frame No Error {
                                }
                                frame Error {
                                n291 = Delete From Array(array=w437, length=1 ("长度"), index=2 ("索引")) -> (array with subset deleted=w438:string[])  [unwired: 1 out]
                                n292 = call <vilib>:"Clear Errors.vi"("error in (no error)"=w440) -> ("error out"=w439:errorcluster)  [unwired: 5 in, 1 out]
                                n293 = Unbundle(w431) -> (w430:i64, w418:i64, w423:string, "拉位移内最大压力(N)"=w429:dbl, "最大值下限"=w428:dbl, "最大值上限"=w427:dbl, w426:string, w425:string)
                                n294 = Number To Decimal String(number=w418) -> (decimal integer string=w417:string)  [unwired: 1 in]
                                n295 = Bundle(w430, w418, "拉位移内最大压力(N)"=w429, "最大值下限"=w428, "最大值上限"=w427, w426, w425) -> (w424:T9)  [unwired: 1 in]
                                n296 = Concatenate Strings("WHERE TEST_NAME ='" ("condition"), w423, "'", "AND CODE_ID =" ("condition"), w417) -> (w433:string)
                                n297 = call <vilib>:"DB Tools Update Data.vi"("condition"=w433, "data"=w424, "error in (no error)"=w439, "columns"=w438, "table"=w441, "connection reference"=w422) -> ("error out"=w420:errorcluster, "connection reference out"=w421:T8)  [unwired: 4 in]
                                }
                              }
                            }
                            n298 = call <vilib>:"Simple Error Handler.vi"("error in (no error)"=w396) -> ()  [unwired: 4 in, 5 out]
                          }
                          frame #1 {
                            n299 = shared-variable "我的电脑\\200滑移力曲线.lvlib\\拉压力测试状态"(u16 1003 ("备用1")) -> ()  [unwired: 1 in, 1 out]
                          }
                        }
                      }
                    }
                  }
                  frame 1003 {
                    n300 = global read "Global1.vi" "联机模式"() -> (w443:enum16{"单机", "追溯"})
                    n301 = case shown="\"追溯\"" w443 {
                      tunnel: w443 -> [_ w446]
                      frame "单机", Default {
                        n302 = shared-variable "我的电脑\\200滑移力曲线.lvlib\\拉压力测试状态"(u16 0 ("备用1")) -> ()  [unwired: 1 in, 1 out]
                        n303 = shared-variable "我的电脑\\200滑移力曲线.lvlib\\备用_1"(u16 0 ("备用_1")) -> ()  [unwired: 1 in, 1 out]
                      }
                      frame "追溯" {
                        n304 = stacked-sequence {
                          tunnel: w446 -> [w447 _]
                          frame #0 {
                            n305 = shared-variable "我的电脑\\200滑移力曲线.lvlib\\生产结果"() -> (w449:u16)  [unwired: 1 in, 1 out]
                            n306 = case shown="2" w449 {
                              tunnel: ["" "OK" "NG"] -> w448
                              frame 0, Default {
                              }
                              frame 1 {
                              }
                              frame 2 {
                              }
                            }
                            n307 = Get Date/Time String(date format (0)=enum16{"short", "long", "abbreviated"}."short" ("日期格式(0)"), want seconds? (F)=FALSE ("需要秒？(F)")) -> (date string=w472:string, time string=w473:string)  [unwired: 1 in]
                            n308 = local read "USER_ID"() -> (w451:string)
                            n309 = local read "deviceid"() -> (w468:string)
                            n310 = local read "codeid"() -> (w470:string)
                            n311 = Concatenate Strings(w472, " " ("字符串"), w473) -> (w475:string)
                            n312 = Search and Replace String(replace all?=TRUE ("替换全部？(F)"), input string=w475, search string="/" ("替换字符串(\"\")"), replace string="-" ("替换字符串(\"\")")) -> (result string=w474:string)  [unwired: 4 in, 3 out]
                            n313 = Decimal String To Number(string=w468, default (0L)=i64 0 ("默认(0 I32)")) -> (number=w469:i64)  [unwired: 1 in, 1 out]
                            n314 = Decimal String To Number(string=w451, default (0L)=i64 0 ("默认(0 I32)")) -> (number=w450:i64)  [unwired: 1 in, 1 out]
                            n315 = Decimal String To Number(string=w470, default (0L)=i64 0 ("默认(0 I32)")) -> (number=w471:i64)  [unwired: 1 in, 1 out]
                            n316 = Bundle(w469, w450, w471, w448, "result string"=w474) -> (w466:T10)  [unwired: 1 in]
                            n317 = call "GetSQLstring.vi"("联机模式"=w447) -> ("错误输出"=w463:errorcluster, "连接字符串"=w462:string)  [unwired: 9 in]
                            n318 = Build Array(w466) -> (w467:T11)
                            n319 = call-poly <vilib>:"DB Tools Open Connection.vi"("error in (no error)"=w463, "connection information"=w462) -> ("error out"=w461:errorcluster, "connection reference"=w464:T8)  [unwired: 6 in]
                            n320 = for {
                              tunnel: w467 -> [w483] mode=indexing
                              tunnel: w464 -> [w481]
                              shift-right: [w479] -> w465
                              shift-left: w461 -> [w486]
                              w482 = string[] ["DEVICE_ID", "USER_ID", "CODE_ID", "RESULT_VALUE", "RESULT_TIME"] ("columns")
                              w484 = "Result" ("table")
                              n321 = call <vilib>:"DB Tools Insert Data.vi"("data"=w483, "error in (no error)"=w486, "columns"=w482, "table"=w484, "connection reference"=w481) -> ("error out"=w485:errorcluster, "connection reference out"=w480:T8)  [unwired: 5 in]
                              n322 = case shown="错误" w485 {
                                selector: w485 -> [w487 w508]
                                tunnel: w482 -> [_ w505]
                                tunnel: w480 -> [w488 w495]
                                tunnel: w484 -> [_ w509]
                                tunnel: w483 -> [_ w499]
                                tunnel: [w488 w494] -> _
                                tunnel: [w487 w493] -> w479
                                frame No Error {
                                }
                                frame Error {
                                n323 = Array Subset(array=w505, index=3 ("长度"), length=2 ("索引")) -> (w506:string[])
                                n324 = Unbundle(w499) -> (w490:i64, w491:i64, w498:string, "result string"=w497:string)  [unwired: 1 out]
                                n325 = Bundle(w498, "result string"=w497) -> (w496:cluster{string, "result string":string})  [unwired: 1 in]
                                n326 = Number To Decimal String(number=w491) -> (decimal integer string=w492:string)  [unwired: 1 in]
                                n327 = call <vilib>:"Clear Errors.vi"("error in (no error)"=w508) -> ("error out"=w507:errorcluster)  [unwired: 5 in, 1 out]
                                n328 = Number To Decimal String(number=w490) -> (decimal integer string=w489:string)  [unwired: 1 in]
                                n329 = Concatenate Strings("WHERE CODE_ID =" ("condition"), w492, "AND DEVICE_ID =", w489) -> (w501:string)
                                n330 = call <vilib>:"DB Tools Update Data.vi"("condition"=w501, "data"=w496, "error in (no error)"=w507, "columns"=w506, "table"=w509, "connection reference"=w495) -> ("error out"=w493:errorcluster, "connection reference out"=w494:T8)  [unwired: 4 in]
                                }
                              }
                            }
                            n331 = call <vilib>:"Simple Error Handler.vi"("error in (no error)"=w465) -> ()  [unwired: 4 in, 5 out]
                          }
                          frame #1 {
                            n332 = shared-variable "我的电脑\\200滑移力曲线.lvlib\\拉压力测试状态"(u16 0 ("备用1")) -> ()  [unwired: 1 in, 1 out]
                            n333 = shared-variable "我的电脑\\200滑移力曲线.lvlib\\备用_1"(u16 0 ("备用_1")) -> ()  [unwired: 1 in, 1 out]
                          }
                        }
                      }
                    }
                  }
                  frame 2000 {
                    n334 = stacked-sequence {
                      frame #0 {
                        n335 = Wait (ms)(milliseconds to wait=u32 300 ("等待时间（毫秒）")) -> ()  [unwired: 1 out]
                        n336 = shared-variable "我的电脑\\Global.lvlib\\传感器码"("" ("传感器码")) -> ()  [unwired: 1 in, 1 out]
                      }
                      frame #1 {
                        w518 = "请扫码！" ("通知内容")
                        n337 = call "浮动通知.vi"("通知内容"=w518) -> ()  [unwired: 11 in]
                        n338 = property on="上序状态" class="Bool (严格)"("Colors [4]"=cluster{u32, u32}[] [{11776947, 11776947}, {11776947, 11776947}, {11776947, 11776947}, {11776947, 11776947}]) -> ()  [unwired: 2 in, 2 out]
                        n339 = local write "上序状态显示"("" ("上序状态显示")) -> ()
                        n340 = call "输入框.vi"("提示信息"=w518) -> ("条形码输出"=w517:string)
                        n341 = shared-variable "我的电脑\\Global.lvlib\\传感器码"(w517) -> ()  [unwired: 1 in, 1 out]
                        n342 = shared-variable "我的电脑\\200滑移力曲线.lvlib\\拉压力测试状态"(u16 2001 ("备用1")) -> ()  [unwired: 1 in, 1 out]
                      }
                    }
                  }
                  frame 2001 {
                    n343 = shared-variable "我的电脑\\Global.lvlib\\传感器码"() -> (w521:string)  [unwired: 1 in, 1 out]
                    n344 = String Length(string=w521) -> (length=w520:i32)
                    n345 = Greater?(x=w520, y=4) -> (0:w522:bool)
                    n346 = case shown="真" w522 {
                      frame False {
                      }
                      frame True {
                        n347 = shared-variable "我的电脑\\200滑移力曲线.lvlib\\拉压力测试状态"(u16 2100 ("备用1")) -> ()  [unwired: 1 in, 1 out]
                      }
                    }
                  }
                  frame 2100 {
                    n348 = global read "Global1.vi" "联机模式"() -> (w524:enum16{"单机", "追溯"})
                    n349 = case shown="\"追溯\"" w524 {
                      frame "单机", Default {
                        n350 = shared-variable "我的电脑\\200滑移力曲线.lvlib\\拉压力测试状态"(u16 2002 ("备用1")) -> ()  [unwired: 1 in, 1 out]
                      }
                      frame "追溯" {
                        n351 = stacked-sequence {
                          frame #0 {
                            n352 = shared-variable "我的电脑\\Global.lvlib\\传感器码"() -> (w527:string)  [unwired: 1 in, 1 out]
                            n353 = local read "productid"() -> (w529:string)
                            n354 = global read "Global1.vi" "联机模式"() -> (w547:enum16{"单机", "追溯"})
                            n355 = call "GetSQLstring.vi"("联机模式"=w547) -> ("错误输出"=w545:errorcluster, "连接字符串"=w546:string)  [unwired: 9 in]
                            n356 = Concatenate Strings("SELECT CODE_ID  FROM CODE  WHERE CODE_SENSOR ='" ("字符串"), w527, "'" ("字符串"), " AND PRODUCT_ID='" ("字符串"), w529, "'" ("字符串")) -> (w544:string)
                            n357 = call-poly <vilib>:"DB Tools Open Connection.vi"("error in (no error)"=w545, "connection information"=w546) -> ("error out"=w538:errorcluster, "connection reference"=w539:T8)  [unwired: 6 in]
                            n358 = call-poly <vilib>:"DB Tools Execute Query.vi"("error in (no error)"=w538, "SQL query"=w544, "connection reference"=w539) -> ("error out"=w542:errorcluster, "recordset reference"=w543:T12)  [unwired: 5 in]
                            n359 = call-poly <vilib>:"DB Tools Fetch Recordset Data.vi"("error in (no error)"=w542, "recordset reference"=w543) -> ("error out"=w537:errorcluster, "recordset data"=w541:variant[][])  [unwired: 3 in, 1 out]
                            n360 = Variant To Data(error in=w537, type=string[][] [], Variant=w541) -> (data=w536:string[][])  [unwired: 1 out]
                            n361 = Index Array(array=w536, index (row)=0 ("索引 (行)")) -> (element=w534:string[])  [unwired: 1 in]
                            n362 = Index Array(array=w534, index=0 ("索引 (行)")) -> (element=w532:string)
                            n363 = local write "codeid"(w532) -> ()
                          }
                          frame #1 {
                            n364 = local read "Fdeviceid"() -> (w548:string)
                            n365 = global read "Global1.vi" "联机模式"() -> (w568:enum16{"单机", "追溯"})
                            n366 = local read "codeid"() -> (w550:string)
                            n367 = call "GetSQLstring.vi"("联机模式"=w568) -> ("错误输出"=w566:errorcluster, "连接字符串"=w567:string)  [unwired: 9 in]
                            n368 = Concatenate Strings("SELECT RESULT_VALUE FROM RESULT  WHERE DEVICE_ID =\n" ("table"), w548, " AND CODE_ID ='" ("字符串"), w550, "'" ("字符串")) -> (w565:string)
                            n369 = call-poly <vilib>:"DB Tools Open Connection.vi"("error in (no error)"=w566, "connection information"=w567) -> ("error out"=w559:errorcluster, "connection reference"=w560:T8)  [unwired: 6 in]
                            n370 = call-poly <vilib>:"DB Tools Execute Query.vi"("error in (no error)"=w559, "SQL query"=w565, "connection reference"=w560) -> ("error out"=w563:errorcluster, "recordset reference"=w564:T12)  [unwired: 5 in]
                            n371 = call-poly <vilib>:"DB Tools Fetch Recordset Data.vi"("error in (no error)"=w563, "recordset reference"=w564) -> ("error out"=w557:errorcluster, "recordset data"=w562:variant[][])  [unwired: 3 in, 1 out]
                            n372 = Variant To Data(error in=w557, type=string[][] [], Variant=w562) -> (data=w553:string[][])  [unwired: 1 out]
                            n373 = Index Array(array=w553, index (row)=0 ("索引 (行)")) -> (element=w555:string[])  [unwired: 1 in]
                            n374 = Index Array(array=w555, index=0 ("索引 (行)")) -> (element=w552:string)
                            n375 = case shown="\"NG\"" w552 {
                              frame "假", Default {
                              }
                              frame "" {
                                n376 = shared-variable "我的电脑\\200滑移力曲线.lvlib\\拉压力测试状态"(u16 5000 ("备用1")) -> ()  [unwired: 1 in, 1 out]
                                n377 = property on="上序状态" class="Bool (严格)"("Colors [4]"=cluster{u32, u32}[] [{16767232, 16767232}, {16767232, 16767232}, {16767232, 16767232}, {16767232, 16767232}]) -> ()  [unwired: 2 in, 2 out]
                                n378 = local write "上序状态显示"("漏序" ("上序状态显示")) -> ()
                              }
                              frame "OK" {
                                n379 = shared-variable "我的电脑\\200滑移力曲线.lvlib\\拉压力测试状态"(u16 2002 ("备用1")) -> ()  [unwired: 1 in, 1 out]
                                n380 = property on="上序状态" class="Bool (严格)"("Colors [4]"=cluster{u32, u32}[] [{6618880, 6618880}, {6618880, 6618880}, {6618880, 6618880}, {6618880, 6618880}]) -> ()  [unwired: 2 in, 2 out]
                                n381 = local write "上序状态显示"("合格" ("上序状态显示")) -> ()
                              }
                              frame "NG" {
                                n382 = shared-variable "我的电脑\\200滑移力曲线.lvlib\\拉压力测试状态"(u16 5000 ("备用1")) -> ()  [unwired: 1 in, 1 out]
                                n383 = property on="上序状态" class="Bool (严格)"("Colors [4]"=cluster{u32, u32}[] [{16711680, 16711680}, {16711680, 16711680}, {16711680, 16711680}, {16711680, 16711680}]) -> ()  [unwired: 2 in, 2 out]
                                n384 = local write "上序状态显示"("不合格" ("上序状态显示")) -> ()
                              }
                            }
                          }
                        }
                      }
                    }
                  }
                }
              }
            }
            n385 = shared-variable "我的电脑\\Global.lvlib\\传感器码"() -> (→"产品追溯码":string)  [unwired: 1 in, 1 out]
          }
          event "删除": Value Change {
            n386 = event-data() -> ("NewVal"=w578:bool)  [unwired: 1 in, 5 out]
            n387 = case shown="真" w578 {
              tunnel: w579 -> [_ w581]
              frame False {
              }
              frame True {
                n388 = Concatenate Strings("确认删除“", "请选择要删除的产品", "”吗？") -> (w583:string)
                n389 = Two Button Dialog(message=w583) -> (T button?=w582:bool)  [unwired: 2 in]
                n390 = case shown="真" w582 {
                  tunnel: w581 -> [_ w587]
                  tunnel: "请选择要删除的产品" -> [_ w586]
                  frame False {
                  }
                  frame True {
                    n391 = call <vilib>:"Open Config Data.vi"("configuration file path"=w587) -> ("error out"=w589:errorcluster, "refnum"=w592:T4)  [unwired: 8 in, 1 out]
                    n392 = call <vilib>:"Remove Section.vi"("section"=w586, "error in (no error)"=w589, "refnum"=w592) -> ("error out"=w591:errorcluster, "section exists?"=w588:bool, "refnum out"=w590:T4)  [unwired: 6 in]
                    n393 = case shown="假" w588 {
                      frame False {
                        n394 = One Button Dialog(message="删除失败！\n请确认产品存在！" ("消息")) -> ()  [unwired: 1 in, 1 out]
                      }
                      frame True {
                        n395 = One Button Dialog(message="删除成功！" ("消息")) -> ()  [unwired: 1 in, 1 out]
                      }
                    }
                    n396 = call <vilib>:"Close Config Data.vi"("error in (no error)"=w591, "refnum"=w590) -> ()  [unwired: 8 in, 2 out]
                  }
                }
              }
            }
          }
          event "确定": Value Change {
            n397 = event-data() -> ("NewVal"=w595:bool)  [unwired: 1 in, 5 out]
            n398 = case shown="真" w595 {
              frame False {
              }
              frame True {
                n399 = stacked-sequence {
                  seq-local: [w599 _ _ _ _ _ _] -> [_ _ _ _ _ _ _]
                  frame #0 {
                    n400 = global read "Global1.vi" "联机模式"() -> (w596:enum16{"单机", "追溯"})
                    n401 = case shown="\"追溯\"" w596 {
                      frame "单机", Default {
                      }
                      frame "追溯" {
                        n402 = local read "产品型号"() -> (w606:string)
                        n403 = call "Get_Device_ID.vi"() -> ("Device_ID"=→"deviceid":string)  [unwired: 10 in, 1 out]
                        n404 = call "GET_PRODUCT_ID.vi"("PRODFUCT_NAME"=w606) -> ("PRODUCT_ID"=w605:string)  [unwired: 10 in]
                        "productid" <- w605
                        n405 = call "查询前序设备.vi"("PRODUCT_ID"=w605) -> ("前序工位"=w604:string[])  [unwired: 10 in]
                        n406 = Index Array(array=w604, index=0 ("索引")) -> (element=→"Fdeviceid":string)
                      }
                    }
                    n407 = local read "产品型号"() -> (w598:string)
                    "产品型号" <- w598
                    n408 = shared-variable "我的电脑\\Global.lvlib\\产品型号"(w598) -> ()  [unwired: 1 in, 1 out]
                    n409 = String Subset(string=w598, offset (0)=u16 2 ("偏移量(0)"), length (rest)=u16 4 ("长度（剩余）")) -> (substring=w599:string)
                    n410 = property on="选项卡控件 2" class="TabCtl (严格)"("Value"=enum32{"滑移力曲线", "参数查看"}."滑移力曲线" ("选项卡控件 2")) -> ()  [unwired: 2 in, 2 out]
                    n411 = Fract/Exp String To Number(string=w599) -> ()  [unwired: 3 in, 2 out]
                  }
                  frame #1 {
                    n412 = local read "用户名"() -> (w609:string)
                    n413 = global read "Global1.vi" "联机模式"() -> (w615:enum16{"单机", "追溯"})
                    n414 = call "GetSQLstring.vi"("联机模式"=w615) -> ("错误输出"=w617:errorcluster, "连接字符串"=w616:string)  [unwired: 9 in]
                    n415 = call-poly <vilib>:"DB Tools Open Connection.vi"("error in (no error)"=w617, "connection information"=w616) -> ("error out"=w623:errorcluster, "connection reference"=w622:T8)  [unwired: 6 in]
                    n416 = Concatenate Strings("SELECT USER_ID FROM [User]  WHERE USER_NAME ='", w609, "'" ("字符串")) -> (w618:string)
                    n417 = call-poly <vilib>:"DB Tools Execute Query.vi"("error in (no error)"=w623, "SQL query"=w618, "connection reference"=w622) -> ("error out"=w620:errorcluster, "recordset reference"=w619:T12)  [unwired: 5 in]
                    n418 = call-poly <vilib>:"DB Tools Fetch Recordset Data.vi"("error in (no error)"=w620, "recordset reference"=w619) -> ("error out"=w624:errorcluster, "recordset data"=w621:variant[][])  [unwired: 3 in, 1 out]
                    n419 = Variant To Data(error in=w624, type=string[][] [], Variant=w621) -> (data=w625:string[][])  [unwired: 1 out]
                    n420 = Index Array(array=w625, index (row)=0 ("索引 (行)")) -> (element=w626:string[])  [unwired: 1 in]
                    n421 = Index Array(array=w626, index=0 ("索引 (行)")) -> (element=→"USER_ID":string)
                  }
                  frame #2 {
                    n422 = local read "坐标轴参数"() -> (w631:string[][])
                    n423 = Index Array(array=w631, index (row) #1=0 ("索引 (行)"), index (row) #2=1 ("索引 (行)"), index (row) #3=2 ("索引 (行)"), index (row) #4=3 ("索引 (行)")) -> (element #1=w643:string[], element #2=w638:string[], element #3=w637:string[], element #4=w636:string[])  [unwired: 4 in]
                    n424 = Index Array(array=w643, index=1 ("索引")) -> (element=w635:string)
                    n425 = Index Array(array=w638, index=1 ("索引")) -> (element=w634:string)
                    n426 = Index Array(array=w637, index=1 ("索引")) -> (element=w633:string)
                    n427 = Index Array(array=w636, index=1 ("索引")) -> (element=w632:string)
                    n428 = Fract/Exp String To Number(string=w635) -> (number=w630:dbl)  [unwired: 3 in, 1 out]
                    n429 = Fract/Exp String To Number(string=w634) -> (number=w629:dbl)  [unwired: 3 in, 1 out]
                    n430 = Fract/Exp String To Number(string=w633) -> (number=w628:dbl)  [unwired: 3 in, 1 out]
                    n431 = Fract/Exp String To Number(string=w632) -> (number=w627:dbl)  [unwired: 3 in, 1 out]
                    n432 = property on="力位移曲线 3" class="XYGraph (严格)"("XScale.Minimum"=w630) -> ()  [unwired: 2 in, 2 out]
                    n433 = property on="力位移曲线 3" class="XYGraph (严格)"("XScale.Maximum"=w629) -> ()  [unwired: 2 in, 2 out]
                    n434 = property on="力位移曲线 3" class="XYGraph (严格)"("YScale.Minimum"=w628) -> ()  [unwired: 2 in, 2 out]
                    n435 = property on="力位移曲线 3" class="XYGraph (严格)"("YScale.Maximum"=w627) -> ()  [unwired: 2 in, 2 out]
                  }
                  frame #3 {
                    n436 = local read "判定框参数"() -> (w657:string[][])
                    n437 = Index Array(array=w657, index (row) #1=0 ("索引 (行)"), index (row) #2=1 ("索引 (行)"), index (row) #3=2 ("索引 (行)"), index (row) #4=3 ("索引 (行)")) -> (element #1=w665:string[], element #2=w660:string[], element #3=w659:string[], element #4=w658:string[])  [unwired: 4 in]
                    n438 = Index Array(array=w665, index=1 ("索引")) -> (element=w652:string)
                    n439 = Index Array(array=w660, index=1 ("索引")) -> (element=w651:string)
                    n440 = Index Array(array=w659, index=1 ("索引")) -> (element=w650:string)
                    n441 = Index Array(array=w658, index=1 ("索引")) -> (element=w649:string)
                    n442 = local read "力位移曲线 3"() -> (w670:cluster{dbl[], dbl[]}[])
                    n443 = Fract/Exp String To Number(string=w652) -> (number=w656:dbl)  [unwired: 3 in, 1 out]
                    n444 = Fract/Exp String To Number(string=w651) -> (number=w655:dbl)  [unwired: 3 in, 1 out]
                    n445 = Fract/Exp String To Number(string=w650) -> (number=w653:dbl)  [unwired: 3 in, 1 out]
                    n446 = Fract/Exp String To Number(string=w649) -> (number=w654:dbl)  [unwired: 3 in, 1 out]
                    n447 = for {
                      tunnel: [w677] -> w648 mode=indexing
                      tunnel: w670 -> [w676] mode=indexing
                      tunnel: w656 -> [w674]
                      tunnel: w655 -> [w673]
                      tunnel: w654 -> [w672]
                      tunnel: w653 -> [w671]
                      i -> [w675]
                      n448 = case shown="0" w675 {
                        tunnel: [w678 w683] -> w677
                        tunnel: w676 -> [w678 _]
                        tunnel: w674 -> [_ w682]
                        tunnel: w673 -> [_ w681]
                        tunnel: w672 -> [_ w680]
                        tunnel: w671 -> [_ w679]
                        frame Default {
                        }
                        frame 0 {
                          n449 = Build Array(w682, w682, w681, w681, w682) -> (w684:dbl[])
                          n450 = Build Array(w679, w680, w680, w679, w679) -> (w685:dbl[])
                          n451 = Bundle(w684, w685) -> (w683:cluster{dbl[], dbl[]})  [unwired: 1 in]
                        }
                      }
                    }
                    n452 = local write "力位移曲线 3"(w648) -> ()
                  }
                  frame #4 {
                    n453 = local read "判定框参数"() -> (w686:string[][])
                    n454 = Index Array(array=w686, index (row) #1=4 ("索引 (行)"), index (row) #2=5 ("索引 (行)"), index (row) #3=6 ("索引 (行)"), index (row) #4=7 ("索引 (行)")) -> (element #1=w704:string[], element #2=w699:string[], element #3=w698:string[], element #4=w697:string[])  [unwired: 4 in]
                    n455 = Index Array(array=w704, index=1 ("索引")) -> (element=w692:string)
                    n456 = Index Array(array=w699, index=1 ("索引")) -> (element=w691:string)
                    n457 = Index Array(array=w698, index=1 ("索引")) -> (element=w690:string)
                    n458 = Index Array(array=w697, index=1 ("索引")) -> (element=w689:string)
                    n459 = local read "力位移曲线 3"() -> (w687:cluster{dbl[], dbl[]}[])
                    n460 = Fract/Exp String To Number(string=w692) -> (number=w696:dbl)  [unwired: 3 in, 1 out]
                    n461 = Fract/Exp String To Number(string=w691) -> (number=w695:dbl)  [unwired: 3 in, 1 out]
                    n462 = Fract/Exp String To Number(string=w690) -> (number=w693:dbl)  [unwired: 3 in, 1 out]
                    n463 = Fract/Exp String To Number(string=w689) -> (number=w694:dbl)  [unwired: 3 in, 1 out]
                    n464 = for {
                      tunnel: [w715] -> w688 mode=indexing
                      tunnel: w687 -> [w714] mode=indexing
                      tunnel: w696 -> [w712]
                      tunnel: w695 -> [w711]
                      tunnel: w694 -> [w710]
                      tunnel: w693 -> [w709]
                      i -> [w713]
                      n465 = case shown="1" w713 {
                        tunnel: [w716 w721] -> w715
                        tunnel: w714 -> [w716 _]
                        tunnel: w712 -> [_ w720]
                        tunnel: w711 -> [_ w719]
                        tunnel: w710 -> [_ w718]
                        tunnel: w709 -> [_ w717]
                        frame Default {
                        }
                        frame 1 {
                          n466 = Build Array(w720, w720, w719, w719, w720) -> (w722:dbl[])
                          n467 = Build Array(w717, w718, w718, w717, w717) -> (w723:dbl[])
                          n468 = Bundle(w722, w723) -> (w721:cluster{dbl[], dbl[]})  [unwired: 1 in]
                        }
                      }
                    }
                    n469 = local write "力位移曲线 3"(w688) -> ()
                  }
                  frame #5 {
                    n470 = local read "结果判定参数"() -> (w736:string[][])
                    n471 = Index Array(array=w736, index (row) #1=0 ("索引 (行)"), index (row) #2=0 ("索引 (行)"), index (row) #3=1 ("索引 (行)"), index (row) #4=1 ("索引 (行)")) -> (element #1=w744:string[], element #2=w743:string[], element #3=w742:string[], element #4=w741:string[])  [unwired: 4 in]
                    n472 = Index Array(array=w744, index=1 ("索引")) -> (element=w740:string)
                    n473 = Index Array(array=w743, index=2 ("索引")) -> (element=w739:string)
                    n474 = Index Array(array=w742, index=1 ("索引")) -> (element=w738:string)
                    n475 = Index Array(array=w741, index=2 ("索引")) -> (element=w737:string)
                    n476 = Fract/Exp String To Number(string=w740) -> (number=→"最大值上限":dbl)  [unwired: 3 in, 1 out]
                    n477 = Fract/Exp String To Number(string=w739) -> (number=→"最大值下限":dbl)  [unwired: 3 in, 1 out]
                    n478 = Fract/Exp String To Number(string=w738) -> (number=→"最小值上限":dbl)  [unwired: 3 in, 1 out]
                    n479 = Fract/Exp String To Number(string=w737) -> (number=→"最小值下限":dbl)  [unwired: 3 in, 1 out]
                  }
                  frame #6 {
                    w745 = "参数装载成功！" ("消息")
                    n480 = call "浮动通知.vi"("通知内容"=w745) -> ()  [unwired: 11 in]
                    n481 = One Button Dialog(message=w745) -> ()  [unwired: 1 in, 1 out]
                  }
                }
              }
            }
          }
          event "添加": Value Change {
            n482 = event-data() -> ("NewVal"=w748:bool)  [unwired: 1 in, 5 out]
            n483 = local read "请输入添加的产品名称"() -> (w749:string)
            n484 = call <vilib>:"Trim Whitespace.vi"("string"=w749) -> ("trimmed string"=w750:string)  [unwired: 1 in]
            n485 = White Space?(1:w750) -> (0:w751:bool)
            n486 = case shown="假" w751 {
              tunnel: w746 -> [w754 _]
              tunnel: w748 -> [w753 _]
              tunnel: w747 -> [w752 _]
              frame False {
                n487 = case shown="真" w753 {
                  tunnel: w754 -> [_ w756]
                  tunnel: w752 -> [_ w755]
                  frame False {
                  }
                  frame True {
                    n488 = for {
                      tunnel: w756 -> [w759] mode=indexing
                      tunnel: w755 -> [w758]
                      n489 = call "Read_Write ParaINI File.vi"("Mode"=enum16{"Read", "Write"}."Write", "Section"="请输入添加的产品名称", "Filepath"=w758, "Ctl Refnum"=w759) -> ()  [unwired: 7 in, 1 out]
                    }
                  }
                }
              }
              frame True {
                w761 = 64 items=["None"=0, "Hand, Error, Stop"=16, "Question"=32, "Exclamation, Warning"=48, "Asterisk, Information"=64] ("icon")
                w762 = 0 items=["OK", "OKCancel", "AbortRetryIgnore", "YesNoCancel", "YesNo", "RetryCancel"] ("buttons")
                n490 = call "信息框（标题、文本、图标）.vi"("icon"=w761, "buttons"=w762, "caption"="添加失败", "text"="请输入产品名称!") -> ()  [unwired: 6 in, 2 out]
              }
            }
          }
          event "产品型号": Value Change {
            n491 = event-data() -> ()  [unwired: 1 in, 6 out]
            n492 = stacked-sequence {
              tunnel: w765 -> [_ w768]
              tunnel: w766 -> [_ w767]
              frame #0 {
              }
              frame #1 {
                n493 = for {
                  tunnel: w768 -> [w771] mode=indexing
                  tunnel: w767 -> [w770]
                  n494 = local read "产品型号"() -> (w769:string)
                  n495 = call "Read_Write ParaINI File.vi"("Mode"=enum16{"Read", "Write"}."Read", "Section"=w769, "Filepath"=w770, "Ctl Refnum"=w771) -> ()  [unwired: 7 in, 1 out]
                }
              }
            }
          }
          event "退出": Value Change {
            n496 = event-data() -> ()  [unwired: 1 in, 6 out]
            n497 = control-ref of="本VI"() -> (w775:refnum<vi>)
            n498 = invoke class="VI" method="FP.Close"(reference=w775) -> (reference out=w773:refnum<vi>, error out=w774:errorcluster)  [unwired: 2 in, 1 out]
            n499 = Close Reference(reference=w773, error in (no error)=w774) -> ()  [unwired: 1 out]
          }
          event "更新": Value Change {
            n500 = event-data() -> ("NewVal"=w778:bool)  [unwired: 1 in, 5 out]
            n501 = case shown="真" w778 {
              tunnel: w777 -> [_ w781]
              tunnel: w776 -> [_ w780]
              frame False {
              }
              frame True {
                n502 = for {
                  tunnel: w781 -> [w786]
                  tunnel: w780 -> [w785] mode=indexing
                  tunnel: [w784] -> w779
                  n503 = local read "产品型号"() -> (w788:string)
                  n504 = call "Read_Write ParaINI File.vi"("Mode"=enum16{"Read", "Write"}."Write", "Section"=w788, "Filepath"=w786, "Ctl Refnum"=w785) -> ("error out"=w784:errorcluster)  [unwired: 7 in]
                }
                n505 = case shown="无错误" w779 {
                  frame No Error {
                    n506 = call "浮动通知.vi"("通知内容"="更新成功！") -> ()  [unwired: 11 in]
                  }
                  frame Error {
                    n507 = call "浮动通知.vi"("通知内容"="更新失败！") -> ()  [unwired: 11 in]
                  }
                }
              }
            }
          }
          event "请输入添加的产品名称": Value Change {
            n508 = event-data() -> ("NewVal"=w789:string)  [unwired: 1 in, 5 out]
            n509 = control-ref of="产品型号"() -> (w790:refnum<vi>)
            n510 = property on="属性节点" class="CmbBox"(reference=w790) -> ("Strings[]"=w791:string[])  [unwired: 1 in, 2 out]
            n511 = for {
              tunnel: w789 -> [w792]
              tunnel: w791 -> [w793] mode=indexing
              n512 = Equal?(x=w792, y=w793) -> (x = y?=w794:bool)
              n513 = case shown="真" w794 {
                tunnel: w792 -> [_ w795]
                frame False {
                }
                frame True {
                  n514 = stacked-sequence {
                    tunnel: w795 -> [w801 _]
                    frame #0 {
                      w796 = 64 items=["None"=0, "Hand, Error, Stop"=16, "Question"=32, "Exclamation, Warning"=48, "Asterisk, Information"=64] ("icon")
                      w797 = 0 items=["OK", "OKCancel", "AbortRetryIgnore", "YesNoCancel", "YesNo", "RetryCancel"] ("buttons")
                      n515 = Concatenate Strings("已经存在产品”" ("text"), w801, "“\n请勿重复添加！" ("字符串")) -> (w799:string)
                      n516 = call "信息框（标题、文本、图标）.vi"("icon"=w796, "buttons"=w797, "caption"="产品重复", "text"=w799) -> ()  [unwired: 6 in, 2 out]
                    }
                    frame #1 {
                      n517 = local write "请输入添加的产品名称"("" ("请输入添加的产品名称")) -> ()
                    }
                  }
                }
              }
            }
          }
          event Panel Close? {
            n518 = event-data() -> ()  [unwired: 1 in, 4 out]
            n519 = control-ref of="本VI"() -> (w809:refnum<vi>)
            n520 = vi-ref "client.vi"() -> (w804:refnum<vi>)
            n521 = invoke class="VI" method="FP.Close"(reference=w809) -> (reference out=w807:refnum<vi>, error out=w808:errorcluster)  [unwired: 2 in, 1 out]
            n522 = invoke class="VI" method="FP.Close"(reference=w804) -> (reference out=w805:refnum<vi>, error out=w806:errorcluster)  [unwired: 2 in, 1 out]
            n523 = Close Reference(reference=w807, error in (no error)=w808) -> ()  [unwired: 1 out]
            n524 = Close Reference(reference=w805, error in (no error)=w806) -> ()  [unwired: 1 out]
            n525 = global write "Global.vi" "程序关闭"(TRUE ("程序关闭")) -> ()
            n526 = event-data("Discard?"=TRUE ("放弃？")) -> ()  [unwired: 1 in, 1 out]
          }
          event "进入用户管理": Value Change {
            n527 = event-data() -> ()  [unwired: 1 in, 6 out]
            n528 = vi-ref "User_manager.vi"() -> (w813:refnum<vi>)
            n529 = call "CallVI.vi"("VI引用"=w813, "状态"=T1."Maximized") -> ()  [unwired: 11 in, 3 out]
          }
          event "设备故障": Value Change {
            n530 = event-data() -> ()  [unwired: 1 in, 6 out]
            n531 = call "状态改变.vi"("设备状态"=enum16{"设备离线", "设备正常", "设备缺料", "设备故障", "质量报警"}."设备故障") -> ()  [unwired: 11 in]
          }
          event "设备缺料": Value Change {
            n532 = event-data() -> ()  [unwired: 1 in, 6 out]
            n533 = call "状态改变.vi"("设备状态"=enum16{"设备离线", "设备正常", "设备缺料", "设备故障", "质量报警"}."设备缺料") -> ()  [unwired: 11 in]
          }
          event "质量报警": Value Change {
            n534 = event-data() -> ()  [unwired: 1 in, 6 out]
            n535 = call "状态改变.vi"("设备状态"=enum16{"设备离线", "设备正常", "设备缺料", "设备故障", "质量报警"}."质量报警") -> ()  [unwired: 11 in]
          }
        }
        n536 = global read "Global.vi" "程序关闭"() -> (w113:bool)
      }
    }
  }
